vi "PECT - Scan no trigger - Autonics - each line.vi"() -> ()   [LabVIEW 2018]
uses:
  <vilib>/DAQmx/configure/timing.llb/DAQmx Timing (Sample Clock).vi
  <resource>/objmgr/daqmx.rc
  <vilib>/measure/NI_MABase.lvlib
  <vilib>/express/express analysis/Spectral/XNode/ExpressSpectralMeasurementsBlockNode.xnode
  <vilib>/express/express analysis/Spectral/Block/exnSpectralBlock spectral measurements PSD poly.vi
  <vilib>/Platform/NI_3dgraph.lvlib
  <vilib>/Instr/_visa.llb/VISA Configure Serial Port (Instr).vi
  <vilib>/Analysis/3filter.llb/Filter Passband Type.ctl
  <vilib>/Analysis/NI_AALBase.lvlib
  <vilib>/DAQmx/configure/trigger.llb/DAQmx Start Trigger (Digital Edge).vi
  <vilib>/DAQmx/read.llb/DAQmx Read (Counter U32 1Chan 1Samp).vi
  <vilib>/DAQmx/create/channels.llb/DAQmx Create Channel (CI-Count Edges).vi
  <vilib>/DAQmx/create/channels.llb/DAQmx Create Channel (AO-Voltage-Basic).vi
  <vilib>/DAQmx/create/channels.llb/DAQmx Create Channel (AI-Voltage-Basic).vi
  <vilib>/DAQmx/write.llb/DAQmx Write (Analog 1D Wfm NChan NSamp).vi
  <vilib>/DAQmx/read.llb/DAQmx Read (Analog Wfm 1Chan NSamp).vi
  <vilib>/DAQmx/read.llb/DAQmx Read (Analog 1D DBL 1Chan NSamp).vi
  <vilib>/express/express analysis/Spectral/Block/exnSpectralBlock spectral measurements PSD WFM.vi
panel:
  out "Output 2D":dbl[][](array[numeric])
  in  "Open 2":bool
  in  "Simulation":bool
  in  "Stop Scan 4":bool
  out "Record path":path=path "D:/NDTENG/Foerster/ROTOMAT/Software/Roto_1.csv" caption="selected path"
  out "Feature Extraction 2":dbl(graph)=0.021153968958947764
  in  "3D Surface":refnum<k7>(container)
  in  "Stop motor":bool
  out "Out Array":dbl[][](array[numeric])
  in  "Distance_":dbl=500.0
  in  "Right 3":bool
  in  "Left 3":bool
  out "Y line":i32 caption="Y percent"
  in  "Move X":bool
  in  "X-length":dbl=20.0
  in  "Y-length":dbl=20.0
  in  "Step Y":dbl=0.2
  in  "1 Min":dbl=0.4
  in  "2 Max":dbl=6.0
  in  "1  Max":dbl=6.0
  in  "2 Min":dbl=0.4
  in  "1 Rate":dbl=0.2
  in  "2 Rate":dbl=0.4
  in  "Travel per Pulse (mm)":dbl=0.002
  in  "Cur. Pos X":dbl=-33.28 format="%#.4f"
  in  "Cur. Pos Y":dbl=30.0 format="%#.4f"
  in  "Save Speed":bool
  in  "COM Port":refnum<visa-resource-name>="COM4"
  in  "Baud Rate":u32=9600
  in  "Data bits":u16=8 min=5 max=8 step=1
  in  "stop bits":u16(ring)=10 items=["1.0"=10, "1.5"=15, "2.0"=20]
  in  "Parity":u16(ring) items=["None", "Odd", "Even", "Mark", "Space"]
  in  "Stop Scan 2":bool
  in  "Scan 2":bool caption="Scan"
  in  "Move Distance (mm)":dbl=16.64
  in  "Counter":tag="Dev1/ctr0"
  in  "ViewMode Analysis":i32(ring) items=["cwViewXYPlane", "cwViewXZPlane", "cwViewYZPlane", "cwViewUserDefined"]
  in  "Plot style Analysis":i32(ring)=5 items=["cwLine"=1, "cwPoint"=2, "cwLinePoint"=3, "cwHiddenLine"=4, "cwSurface"=5, "cwSurfaceLine"=6, "cwSurfaceNormal"=7, "cwContourLine"=8, "cwSurfaceContour"=9]
  in  "Open":bool
  in  "Save Scan mode":bool caption="Save Process"
  in  "Tab Control 2":T1(tab)
  out "Hall sensors signal":waveform(dbl)[](graph)=[{"t0"=timestamp(3525645621.636764 s since 1904-01-01), "dt"=1.9999999999999944e-06, "Y"=array[2100 elements], "attributes"=variant("NI_ChannelName"=variant(string "Dev1/ai0"), "NI_UnitDescription"=variant(string "Volts"))}, {"t0"=timestamp(3525645621.636764 s since 1904-01-01), "dt"=1.9999999999999944e-06, "Y"=array[2100 elements], "attributes"=variant("NI_ChannelName"=variant(string "Dev1/ai0"), "NI_UnitDescription"=variant(string "Volts"))}]
  out "Feature Extraction":dbl(graph)=0.021153968958947764
  out "Waveform Graph 2":waveform(dbl)[](graph)=[{"t0"=timestamp(0 s since 1904-01-01), "dt"=1.25e-06, "Y"=array[8000 elements]}]
  out "Power spectral density":cluster{"f0":dbl, "df":dbl, "magnitude":dbl[]}[](graph)=[{"f0"=0.0, "df"=238.09523809523876, "magnitude"=[-25.4340272409559, -28.495970805276507, -69.09064054555873, -79.11355871279994, -75.69366097931027, -84.18131507822396, -80.50168881348966, -82.72314293089615, -87.19630499623688, -82.83568021481967, -89.95290866002237, -85.90392585035596, -87.41269111550386, -91.40893948681482, -86.69370819914215, -93.36336146616782, -89.019380476413, -89.73232030153878, -94.58261196624535, -89.16287927388944, -94.965890302584, -91.86846413178648, -91.95327957161693, -97.62687167891286, -91.59993648735762, -97.30685711015555, -93.8350762480425, -93.27921214218685, -99.59438563802183, -93.1824258709588, -98.3113125531512, -95.45425138584356, -94.39327135467576, -100.65352961491782, -94.55889081970952, -99.40788907105079, -97.93617495318924, -96.19517579047603, -103.97036797797732, -96.40295202889732, -99.7036956909043, -99.48760137175819, -97.46192979187015, -106.29271483151813, -97.51447379981207, -99.86179280251669, -100.43811038443037, -97.59011642740829, -105.58363666166275, -99.01126121197593, -101.01575323613292, -101.90167607549864, -98.61952569586691, -106.73670466995647, -99.29976101634999, -101.54959604687718, -105.17330050767885, -100.09392305285375, -109.78264848704497, -100.98914236173123, -101.81665207962125, -105.42358374403365, -99.82880728595141, -107.07330885402075, -101.07712607444097, -101.03780825357597, -107.32811151840846, -101.221643458408, -105.63776326231454, -101.8420593566944, -101.80081629073969, -107.47915505307212, -101.12986632760553, -106.84901404755908, -102.73715610491038, -101.51552854007832, -107.28771371003282, -101.3928633472346, -107.44515355816633, -104.89304864643535, -103.1455098860718, -110.19910428997925, -102.73063833081197, -107.57101838377707, -104.90574568581201, -103.72599931018533, -109.97178587260123, -103.24611921258705, -108.36098023558972, -106.6408311450923, -104.73569536588386, -116.21683530762306, -105.02627439976544, -107.15856030450797, -109.81191038702062, -105.53476822084077, -119.10077766590356, -105.31867536160968, -106.9718410299748, -108.34458911268797, -104.70307996109247, -114.76704583683203, -106.29948298493936, -108.55077108437321, -112.16618350190343, -105.98453547558171, -114.68576835450673, -107.50968901677987, -107.89174277914348, -111.59875709602721, -106.69368240333122, -114.93273233954758, -105.23904516482949, -106.00272331017348, -110.36103151258544, -104.93177986717492, -110.8835476773746, -106.69346348818806, -106.66103973993782, -119.11729839814336, -108.06338160849775, -114.5879267769655, -108.59816838472844, -107.53189260743514, -114.07390818184973, -106.70996756049796, -113.27381274118753, -109.50270539577696, -107.37282420343303, -113.4779718725949, -106.04267666963091, -111.30294425571472, -112.46717993668915, -109.13164915488709, -116.65287200885172, -107.03002573045511, -110.21479040603631, -112.476075561056, -106.97710947409149, -119.42145279296255, -108.3200486628316, -110.46641858585929, -117.16650627564961, -109.73297826697552, -120.31689830731365, -107.19513745371916, -110.66663569403087, -113.30365980039964, -110.01971553524372, -123.68660617105166, -110.8171755739396, -111.11382172813546, -117.76239209582961, -109.49899370205401, -115.22252846498625, -111.1932077339224, -112.38235939086871, -118.22207022901702, -110.6546796895719, -116.97450780644367, -110.82401674194465, -111.96705198878843, -118.28092956599232, -110.5621503678909, -121.25720613496851, -111.98371482341479, -113.27928013246557, -111.96833712758355, -108.56859286664552, -120.32790468431601, -110.82699792221703, -110.79062667340345, -122.65756767769517, -110.48843456045427, -116.8782055296399, -115.43719816168479, -114.47619780315773, -121.42183196132746, -111.60631415727042, -120.68077308056417, -109.35478690141552, -109.03210709352732, -120.6260555904793, -109.47936424950136, -113.33719701518146, -112.88325992990137, -110.99901978536154, -123.19636626521421, -109.09861317900774, -113.33125158106256, -115.35673297389727, -112.77249677632989, -124.61163141716472, -114.68140920359865, -121.89642913325117, -115.47413298424323, -112.82196063671608, -127.87542521315149, -111.54178118788309, -113.6448752704395, -120.76569423868874, -112.98651214877823, -123.18868565400437, -115.41399838634062, -115.46853076016815, -116.40989072804102, -110.69611347288615, -132.23164080331392, -114.76376391429793, -121.7246597336247, -117.46893009589195, -114.01899156779395, -125.22079066032327, -114.59524199183258, -114.50034890537415, -122.9532092227648, -113.72727798159212, -125.65163915514907, -113.4793801211504, -110.4090756414644, -125.63592649005872, -114.22938378193007, -116.74947251106808, -121.60535557984142, -116.79385283402802, -122.44667696630361, -113.43873413563811, -123.28159708694415, -113.92892974938164, -114.01193823589753, -121.62751955742443, -118.76839573694522, -125.52998605097204, -115.19609643487229, -117.49409595176479, -117.08423885198002, -119.48314867245172, -125.01675515413412, -117.92668164142911, -115.55962389856793, -125.63488616674975, -119.11862859365166, -114.78860770332909, -117.18339781294443, -111.18063004722558, -118.31775966044624, -111.6867367949252, -114.57226159377, -119.36541212960576, -113.90245139442648, -132.46343443313128, -120.1282759002165, -121.05279009698619, -118.9115822659523, -121.23280439248342, -116.31914159559688, -127.38829313950257, -117.34673005740623, -115.95249861902771, -114.9301657394146, -123.22361802797445, -110.83274939062106, -116.16624248562111, -116.76753364192771, -113.94454545069023, -122.95736945775944, -118.66755800656253, -129.1462641201204, -116.6351050110328, -117.22529407303742, -123.80212197360244, -115.89792176423389, -114.25823938606595, -125.60467961977515, -114.59958849364433, -121.70071005514421, -118.25968972451209, -114.69929400946009, -123.88209034116528, -115.03869272537257, -117.52034211782204, -115.27990843516797, -117.85366603932033, -125.16865559622727, -118.21960424638507, -119.69008755413566, -117.24640963460672, -114.32867295013791, -119.1576982419508, -122.85495988425586, -116.3373010103401, -114.53730203699834, -115.67017599990201, -127.144321037601, -115.73849102686786, -117.7626163106355, -119.7346592991025, -117.41317517684553, -125.0417974461613, -114.5488949833583, -116.59812516173781, -119.91064563147799, -115.27933218667663, -122.09990513751134, -120.95678574143693, -123.25641714743752, -112.5173710452192, -113.53735878806998, -129.23914933506734, -116.27157269711533, -148.4020512032711, -118.84888216023774, -123.82550527215588, -116.87770979616658, -111.32191810025745, -124.32675905891588, -114.37182733794062, -121.10713785851372, -122.59698730059695, -116.38346694563282, -121.69144349152856, -119.00883142493832, -110.81886738196273, -120.7909830607913, -115.01780448665316, -114.52055121633796, -132.6824191654361, -116.330695115645, -126.4664151018508, -118.32717907779282, -118.7288071595281, -120.42749846140066, -112.53185615773879, -124.26026008984286, -114.24089252048742, -120.00368190003405, -114.71738500842926, -112.92262025927133, -129.21127897188563, -113.5947811765517, -117.80802009651353, -117.0133790103226, -112.19210322760304, -118.17549968071762, -119.3256187825503, -118.84981507334446, -121.39118969751144, -114.64543555194373, -119.84814933224528, -114.09123407848944, -116.22899352170892, -116.41650104077173, -113.70057202673476, -124.52773908304957, -114.87372641784933, -116.11651108221098, -121.68680962246994, -115.78306007961302, -122.22621008657796, -118.81157995182392, -113.9402115821658, -132.636729517989, -114.49554876936634, -119.50980190398928, -123.27410972236837, -118.52851881066383, -122.25212982572599, -117.13947036230024, -120.85005588797962, -118.41526503460501, -117.61788553858068, -126.3872056783977, -114.98198608543298, -119.7789938911847, -120.84873579392627, -114.38831474301695, -153.35954756825245, -113.19505610638078, -114.17454820985151, -127.41069917723112, -114.92677241657191, -125.49053973810628, -113.36382196587914, -119.96785250843519, -122.47388530423243, -116.38671253508838, -120.0905790211523, -119.83326265062107, -117.88168146696918, -122.3132169880757, -115.87324909105399, -125.92003267803432, -113.96860176867415, -114.49156118371398, -127.52634390035722, -115.05967156528004, -126.82020221981517, -117.93643187259194, -116.51163213641807, -119.47551219110167, -119.55225172256931, -116.9512257852571, -122.23153124485954, -120.8368476753637, -121.48473913072222, -115.83122660909913, -135.74260014140523, -116.58358375805423, -118.15236945484727, -119.06674062398864, -115.7844834762477, -125.06111738611818, -114.7801535050972, -115.2696605691888, -123.98656374010793, -119.29025555731172, -118.29146803784099, -119.55696172158135, -118.06884171238352, -127.81587648134607, -120.41730580797976, -123.49626136731604, -112.2147141798107, -116.22555232584983, -132.79419178871254, -119.66964883124663, -117.20946469243259, -118.20939292735417, -115.6951914646649, -129.64892855822356, -114.27056999288617, -120.31005512957381, -117.41846777372632, -115.50158386260813, -124.69777160737624, -115.2892897247205, -123.61522771666871, -113.75248734362687, -113.22999749252833, -129.3490509395313, -116.88137735661701, -116.94110280242681, -119.50244079984806, -119.30521139999144, -128.17199984115797, -118.06736594940236, -116.05331575995922, -121.29670750650897, -116.1140297602044, -125.090619084802, -121.41807296062154, -120.01332757902264, -120.54914530643151, -116.49738633175463, -122.32551291835904, -118.3190808346865, -118.92638453656723, -122.48819531011718, -117.01021725424317, -120.98896352560598, -117.23831688685218, -121.27915259197124, -121.20017251921661, -117.6155648860373, -120.91300272912063, -117.94438460863424, -115.94437430101533, -123.35904829443987, -117.74011174503076, -121.54935745388448, -120.82564553545025, -121.98951430455743, -120.24858103448778, -116.44403527138395, -112.79571494351876, -112.42801913096545, -110.1697573019791, -115.34500457736401, -119.81921052956707, -129.82600951154313, -115.5862301263047, -112.59292882433087, -120.79009137478283, -131.32849293387295, -113.61194478398238, -123.48568856527031, -119.17507777781304, -123.09261867490484, -116.97755217417308, -123.94453461434183, -116.58080525616379, -119.64289646280756, -122.90202645580743, -126.66219093058154, -121.95048829056148, -115.72578023509817, -116.70117814464484, -121.91050280869723, -118.25299095698178, -116.45905559047064, -132.57794493731578, -121.65327820443292, -120.9816664775787, -117.17270262269045, -120.27433984830965, -125.89418976028173, -119.09563505847817, -126.9693215534833, -113.17465524665704, -118.98702092883116, -119.83822568580342, -120.45832738089722, -120.67735960513633, -127.38676010839353, -127.65777338183055, -118.37446329057411, -115.61355494839711, -119.94568688114103, -116.06619937633681, -126.348857777089, -118.92850079147068, -119.5416617639739, -132.47075644221843, -118.08809356028496, -123.16186463092723, -121.51579486791232, -122.88983670053283, -129.5195538417256, -120.4730389608841, -132.16486858341602, -122.34690358436781, -120.71922104337597, -114.29260860841114, -117.67902631803368, -124.7040155514909, -123.51274592117205, -120.02297921674332, -136.54655493811157, -120.45629227407751, -119.06410204276258, -127.91681714792554, -122.82090055753153, -125.16838176650813, -121.79565386970478, -119.79607311590995, -126.54861375039647, -121.59135878113302, -132.8348640697562, -118.1305434733294, -120.46070148841905, -122.69571910896963, -117.6534954653865, -124.15742546824006, -120.73646926947502, -124.82696993800742, -124.513836786494, -123.15395713389651, -124.62395468806395, -117.21365768658171, -119.32635871968456, -121.48532284413152, -119.38242892643675, -126.25575652510352, -123.27133124029851, -117.58533922728374, -118.17710108929799, -114.99496360200965, -117.77133194647278, -111.34898201101595, -111.50817058307922, -119.0703124690998, -127.70676079885351, -121.8704969141074, -125.93154214283446, -118.65628450081473, -122.47918878348962, -117.9651589546518, -126.13560583004508, -122.42294805637847, -133.924453763793, -117.2082573038767, -117.6525335446734, -122.92077297426977, -122.04624645756786, -116.43289028226238, -117.93180959338378, -129.02356734231915, -117.95493621286326, -120.7555929766252, -120.76782849311112, -123.06287498470708, -117.83798593857965, -123.43423215434719, -120.15190119516652, -120.48240443128407, -143.29738987393452, -123.46572247444769, -120.89055325172792, -125.66715973809033, -118.26887578998644, -117.01836200028421, -121.33021830755509, -119.68846363313813, -122.60689066103069, -116.26858138914181, -119.59360791972998, -122.94866175463353, -114.174409515556, -118.00516930888391, -121.56978543579633, -135.87799017759036, -117.50816594504829, -122.82539428457626, -123.82103443155845, -124.77975840345442, -121.13340798086698, -120.93607435603558, -133.15787160745222, -120.70545628137863, -125.02155972441679, -122.04666465472178, -118.01234649746348, -127.88767491042842, -119.02096620167217, -120.16031065152875, -122.25406107859625, -121.72733059051095, -120.61357375519918, -118.63962847172827, -134.3857741605498, -116.3600853185034, -117.26695700691671, -119.9176982185873, -113.45576465218444, -126.69779573632724, -114.39554522802246, -116.8457146515868, -116.34219889483086, -119.30011291548334, -120.01163291843496, -114.29497178248809, -127.65687642749229, -119.58556923753022, -129.8593054181261, -122.2353645100479, -120.79536520223796, -119.83284028355028, -117.7991246185715, -128.390292904734, -119.78079925213122, -125.478913448993, -113.89747777944768, -112.66620124153357, -124.3475049842711, -120.85847303094337, -132.91807981902295, -119.523494985723, -116.65149909866443, -119.73287290436721, -127.63237851524192, -127.23413304048789, -120.87585453904362, -121.08540368080186, -134.91071939669257, -117.75375801669338, -117.2683014590723, -120.9739099492833, -118.23809733632451, -120.94065804928206, -123.88077510875804, -118.13812819300607, -122.60294123365466, -126.97075898006995, -120.18754789731035, -124.71238663441227, -120.55456557278582, -130.94599087480253, -111.18288669417035, -112.27708791831247, -126.0512034600378, -117.41881712783596, -128.20553880273903, -117.29482600885808, -118.2045526390752, -127.81966672699878, -117.03716165902529, -115.46711739757512, -117.15363929234843, -121.87599671671335, -121.19736800869221, -126.5301786755875, -131.20754947382918, -124.40138004810741, -129.0562496906515, -121.06816554587536, -121.01023627802867, -138.6137911215848, -120.12495002524031, -121.38510517514229, -122.79804220535513, -116.97501378195477, -118.82011581137473, -114.0229185604644, -119.54287501990726, -114.64474566771625, -117.76935669872461, -123.81082574158907, -118.51678358865587, -128.9664755188374, -123.45357998434133, -122.74888841574231, -120.74640581234044, -126.956344345126, -119.95682140104577, -118.8873101779055, -124.41062359284174, -128.97304498664363, -123.86287113204068, -127.30257087528216, -120.61364220528216, -114.45119129304715, -119.68384044686806, -131.29639185291157, -122.31250766293485, -119.57420865241102, -124.74014026002448, -124.87593035709094, -118.4566565612952, -123.76236085976001, -120.84780538841838, -117.68987599773281, -135.06195695255914, -122.56143585795171, -129.04610316842883, -118.32313199570537, -117.77093802786419, -124.46572845786741, -129.1123298336903, -120.88470269965448, -116.69988985752187, -116.84054667499878, -133.76883696987278, -122.32434984927302, -124.98940594457933, -122.56515592789917, -118.31562562243366, -133.97049179545627, -122.33220627999802, -131.16753675316977, -124.69828063969263, -116.37621154460467, -126.1833423168025, -129.62937634161355, -118.46241371150788, -117.52851478852457, -125.32425037236442, -119.0327364293772, -124.2861355894013, -123.24573502278234, -125.52155812053758, -113.75743410709823, -114.79513162658353, -128.58142362588052, -122.48277095196701, -118.94747544412269, -123.86988127835491, -124.78140456983323, -121.53998481875398, -116.01432822539552, -119.20174681160661, -122.75167725800814, -120.58657749420254, -118.51141061842183, -119.24457006171983, -131.43641234223372, -116.00759139055087, -121.24442216102587, -123.29371279953725, -117.608355420454, -116.33684374617326, -118.06291688281922, -121.88761866022774, -121.54820313120047, -119.5051369873635, -126.56611158390913, -118.84012713615805, -121.09285296522563, -124.67955377692547, -147.31451139022337, -116.80660421066897, -114.8367853755961, -120.41026468628925, -123.65666101895222, -119.64837119787269, -116.77480172559095, -116.54263359173909, -124.75286620868079, -117.33721912698883, -116.51795620907136, -118.50086748176733, -128.10381328920522, -122.78098994574157, -120.24716756092855, -119.52743204722819, -115.00407387659232, -108.2853711552629, -108.61086943894702, -119.6228894146785, -124.11132022420912, -125.6202218409766, -123.1749360787656, -118.1971196161698, -123.95075368058998, -121.72140109898365, -123.27106899042522, -123.73035629887062, -121.24369679109273, -121.07381526465288, -113.13965659723667, -118.330755475899, -118.40249076804484, -111.59630598649044, -116.1569506845575, -125.67326089915758, -125.85723567111906, -119.24293277595024, -117.87067617433537, -120.70936924059559, -131.8090588468898, -132.98711569625004, -123.63274249467587, -122.75476917502559, -126.12873814250243, -120.53144270605179, -129.07030822919336, -122.7889410422919, -124.35405971166259, -119.63968579420454, -139.0154441054289, -129.47962001806934, -121.86548015410847, -128.6818469257012, -121.40195873232601, -138.64231053781285, -124.22025721762265, -124.06073958736941, -126.71929802352521, -131.7498459276443, -120.68144109742178, -122.6325588818875, -126.80796617875095, -124.92487955227033, -136.94498040498806, -124.26704334219014, -123.21376211221711, -140.25352033075964, -129.53222319772195, -122.58541579060463, -122.1996729592375, -125.66642108013673, -125.66310429236694, -120.09682773706965, -125.27326633941439, -121.55721878725502, -121.22507119941083, -121.53716878624485, -136.20685498111987, -128.15260146013156, -120.03473972471616, -124.60755958763912, -124.73082500077143, -123.93425949983688, -131.04483249265184, -121.7957035014449, -127.09321441816094, -133.6144579272493, -124.69014595896968, -130.4902091211609, -121.18031440773905, -128.00033943961677, -125.88991118115149, -118.865310745079, -123.69668867733147, -117.98756965862728, -114.40013091842827, -118.28685032521078, -122.23464196869948, -124.8440422629961, -129.66281606870848, -119.440534215621, -124.54391783563877, -124.93447967158188, -121.7258558761523, -122.28817885403082, -127.06889620458577, -128.92172974939206, -120.62932166634072, -126.06847321900452, -123.31471168429935, -121.80350826545656, -129.2574604322076, -125.67225933193998, -125.7801671825605, -129.53804733161627, -119.56756644124712, -128.82490314699373, -124.7689736295626, -120.50019729114693, -124.50603158563972, -122.8120627011088, -125.60528875555717, -123.8817354922713, -124.05570537836674, -120.94568834491936, -118.06056028605255, -124.24390361274648, -125.5716703018188, -127.71949519914061, -130.7001652968252, -126.27701412017494, -133.76810134709916, -128.4738939614179, -120.302550881701, -118.91298143662928, -124.9077318110765, -127.16253699189492, -118.11405934812818, -117.52028071290711, -140.95620572748925, -123.61977932545628, -131.0334379970501, -125.88948384968432, -127.81552331993379, -121.92316280719056, -119.05911238768732, -126.83773251459189, -123.52627415002164, -120.8779561023192, -123.66683567603742, -131.64300993967345, -123.62895847772963, -116.89792951363142, -120.1068259250195, -117.92484706459337, -115.58208487778379, -120.76803581628594, -123.95408562090736, -122.79456549632754, -134.5305398779298, -123.57040300991032, -128.40634159414552, -123.70102187824159, -118.24970739397313, -119.66483900349026, -127.78024313111393, -120.3547204111785, -125.49305364308705, -119.49505591004302, -120.50920386196539, -119.03509516851003, -114.24667300009652, -121.60538636584391, -119.95304417598024, -122.24585853682832, -128.63653016912684, -116.04810628805795, -121.94159862131235, -122.59928204398939, -121.4532410501923, -128.6511474663462, -130.83715595958148, -121.71998300574741, -116.91426629511156, -113.587592058512, -115.59736707638731, -124.65300822631244, -133.32538684258748, -124.02289142873636, -121.54278890993639, -119.02596809402394, -108.90572887117857, -112.14974069608851, -129.21149299565423, -118.82148342951197, -116.65510894288538, -118.39609618084175, -116.53502642884725, -122.47549439965209, -122.23125657046063, -123.68081343116663, -120.67915071600007, -123.6899360128769, -118.56721985209728, -118.36641581191942, -126.96724630704657, -119.36877661672403, -123.07698921198843, -117.80772421906035, -122.82545076270567, -118.82755071380888, -117.21030132539394, -129.760567864525, -118.0816708063509, -125.80573274113647, -121.18434666182338, -121.80987210832065, -130.99259828357094, -125.47223579895922, -123.86818606677002, -118.7118158196511, -119.27778317338742, -127.27333258839096, -119.90672352079164, -140.78772370844268, -118.08251080057329, -119.86636232122572, -118.69482489738232, -119.19106512767372, -123.70988914879189, -121.92566832147995, -123.41378261726373, -120.1715186070818, -117.9079629421116, -117.41960207545632, -123.72833996166874, -127.24377206607298, -124.99098647980887, -129.48803701799955, -129.92351350561592, -120.79284154834647, -119.29601975194524, -136.17244775530037, -126.73975437546255, -128.84068276143336, -125.66374985701982, -136.69026010435715, -125.44409235146617, -119.28138070315057, -118.65017329869724, -118.02521532826772, -122.23736063759657, -121.27846943548622, -116.69850478126861, -119.7711336696722, -123.70776561180185, -118.43344549561263, -123.92390877157247, -117.19637143066551, -117.64112988205311, -127.78399195238529]}, ...(2 in all)]
  out "Differential data":dbl[][](graph)
  out "Normal data":dbl[][](graph)
  in  "Emergency Stop":bool
  in  "Stop 3":bool
  in  "Home Y":bool
  in  "Home X":bool
  in  "Back":bool
  in  "Front":bool
  in  "Left":bool
  in  "Right":bool
  in  "Stop Scan":bool
  in  "Scan":bool
  in  "Tab Control":enum32{"     Motor    ", "         DAQ        "}(tab)
  in  "Left_":bool
  in  "Right_":bool
  in  "Home":bool
  in  "Move Distance (mm) 2":dbl=20.0
  in  "Speed":dbl=10.0
  out "Current  Position (mm)":dbl format="%#_4g"
  in  "COM Port 2":refnum<visa-resource-name>="COM3"
  in  "Baud Rate 2":u32=57600
  in  "Stop Scan 3":bool
  in  "Multiplier":dbl=10.0
  in  "Travel per  Pulse":dbl=0.0025
  in  "Low Cutoff Freq":dbl=50.0
  out "Actual Sample Rate":dbl=500000.0 format="%0.2f"
  in  "Physical Channel":tag="Dev5/ai0"
  in  "Min Voltage":dbl=-10.0
  in  "Max Voltage":dbl=10.0
  in  "Terminal Configuration":i32(ring)=10083 items=["default"=-1, "RSE"=10083, "NRSE"=10078, "Differential"=10106, "Pseudodifferential"=12529]
  in  "Sample Clock Source 2":tag="OnboardClock"
  in  "Sample Rate":dbl=500000.0
  out "Number of Samples 2":i32=1000
  out "Actual Sample Rate 2":dbl=800000.0 format="%0.2f"
  in  "Physical Channel(s)":tag="Dev5/ao1"
  in  "Min Voltage 2":dbl=-10.0
  in  "Max Voltage 2":dbl=10.0
  in  "Sample Clock Source":tag="OnboardClock"
  in  "Sample Rate 2":dbl=800000.0
  in  "Number of Samples":i32=8000
  in  "Offset":bool
  in  "2 Plots":bool
  in  "Edge":i32(ring)=10280 items=["Rising"=10280, "Falling"=10171]
  in  "Digital Trigger Source":tag="/Dev5/PFI0"
  in  "Average":i32=10
  in  "Duty cycle %":dbl=50.0 format="%#.2f"
  in  "Stop":bool
  in  "Output Array":T2(array[cluster])=[{"Waveform Type"=2, "Amplitude"=10.0, "Frequency"=1000.0}] {"Frequency" format="%0.2p"; "Amplitude" format="%0.2p"; "Waveform Type" items=["Sine Wave", "Triangle Wave", "Square Wave", "Sawtooth Wave"]}
  # "Pulse Shape"
  # "COM  Setting"
  # "Trigger Settings"
  # "Data Processing"
  # "Speed  Setting"
  # "Scan  Setting"
  # "Pulse"
  # "Hall Sensors Signal"
  # "Feature Extraction"
  # "Power Spectal Density"
  # "COM  Setting"
  # "Scan  Setting"
  # "Pulse  Channel"
  # "Pulse  Timming"
  # "Sensor  Channel"
  # "DAQ Timming"
  # "Logging Settings"
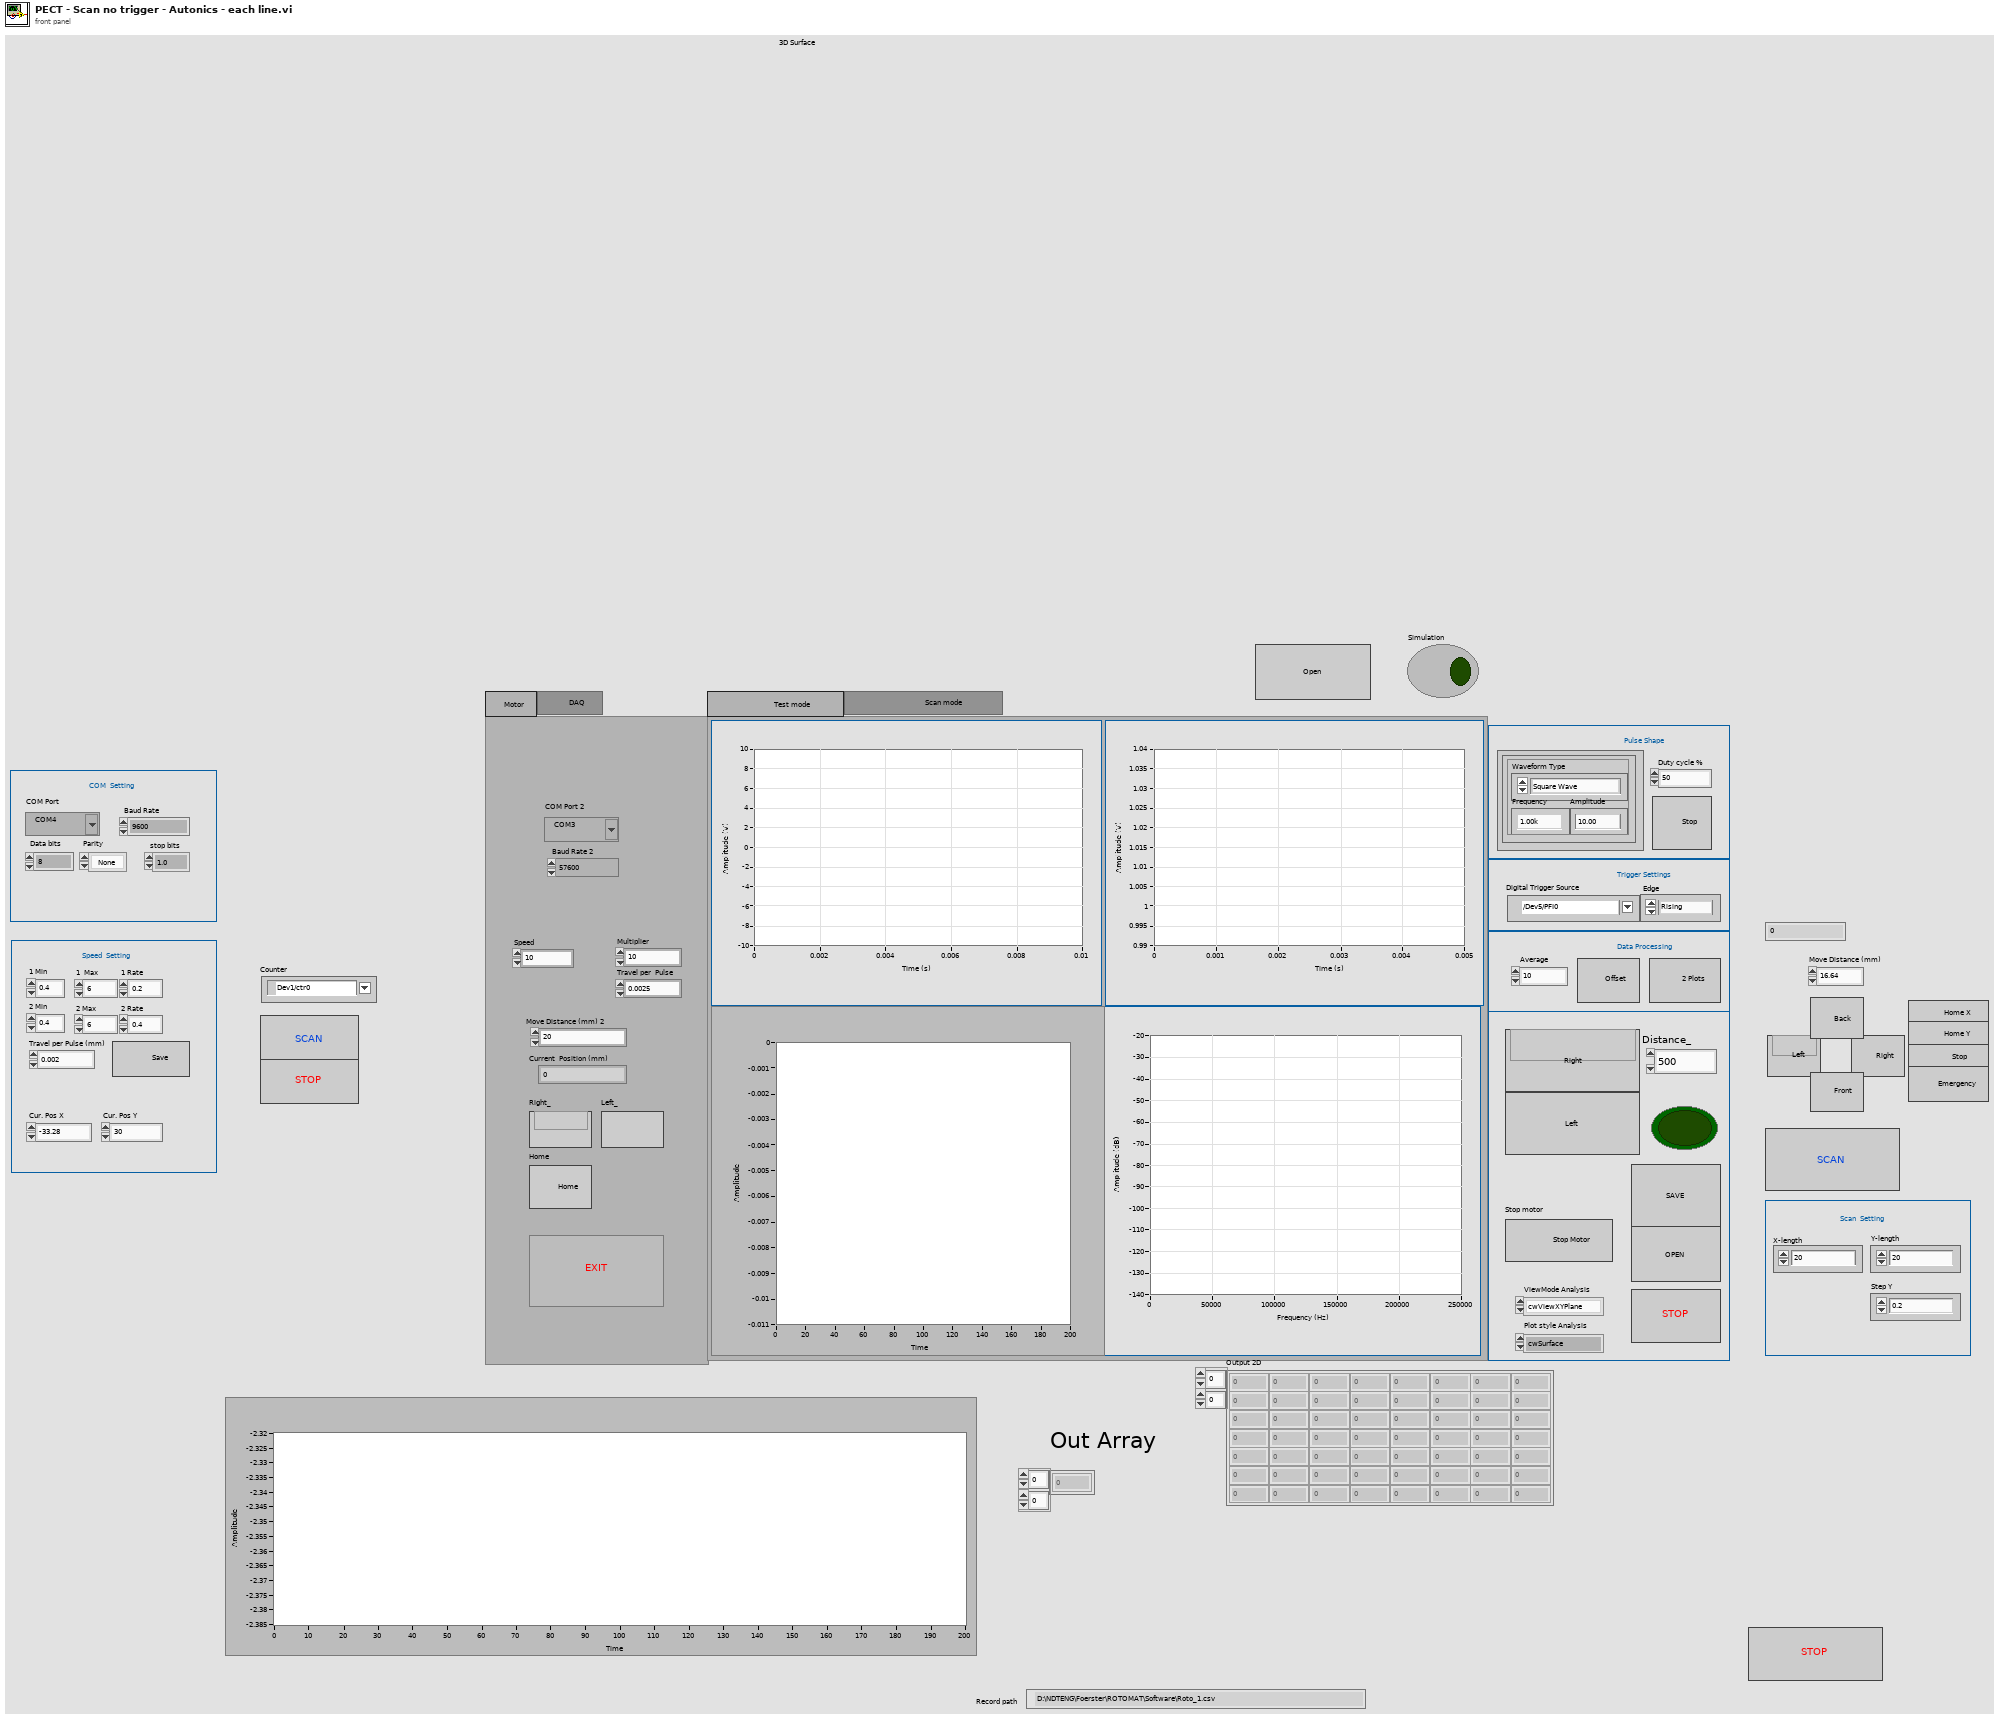
[diagram p1: front panel]
types:
  T1 = enum32{"                    Test mode                   ", "                          Scan mode                      "}
  T2 = cluster{"Waveform Type":u16, "Amplitude":dbl, "Frequency":dbl}[]
  T3 = enum16{"No Scan", "Scan X", "Wait to destination X"}
  T4 = cluster{"Waveform Type":u16, "Amplitude":dbl, "Frequency":dbl}
  T5 = enum16{"open", "open or create", "create or replace", "create", "open (read-only)"}
  T6 = typedef "NI_AALBase.lvlib/Filter Passband Type.ctl" = enum32{"Lowpass", "Highpass", "Bandpass", "Bandstop"}
  T7 = cluster{"averaging mode":u16, "weighting mode":u16, "number of averages":u32}
  T8 = cluster{"dB On (F)":bool, "unwrap phase (F)":bool, "convert to degree (F)":bool}
  T9 = typedef "NI_Matrix.lvlib/RealMatrix.ctl" = dbl[][]
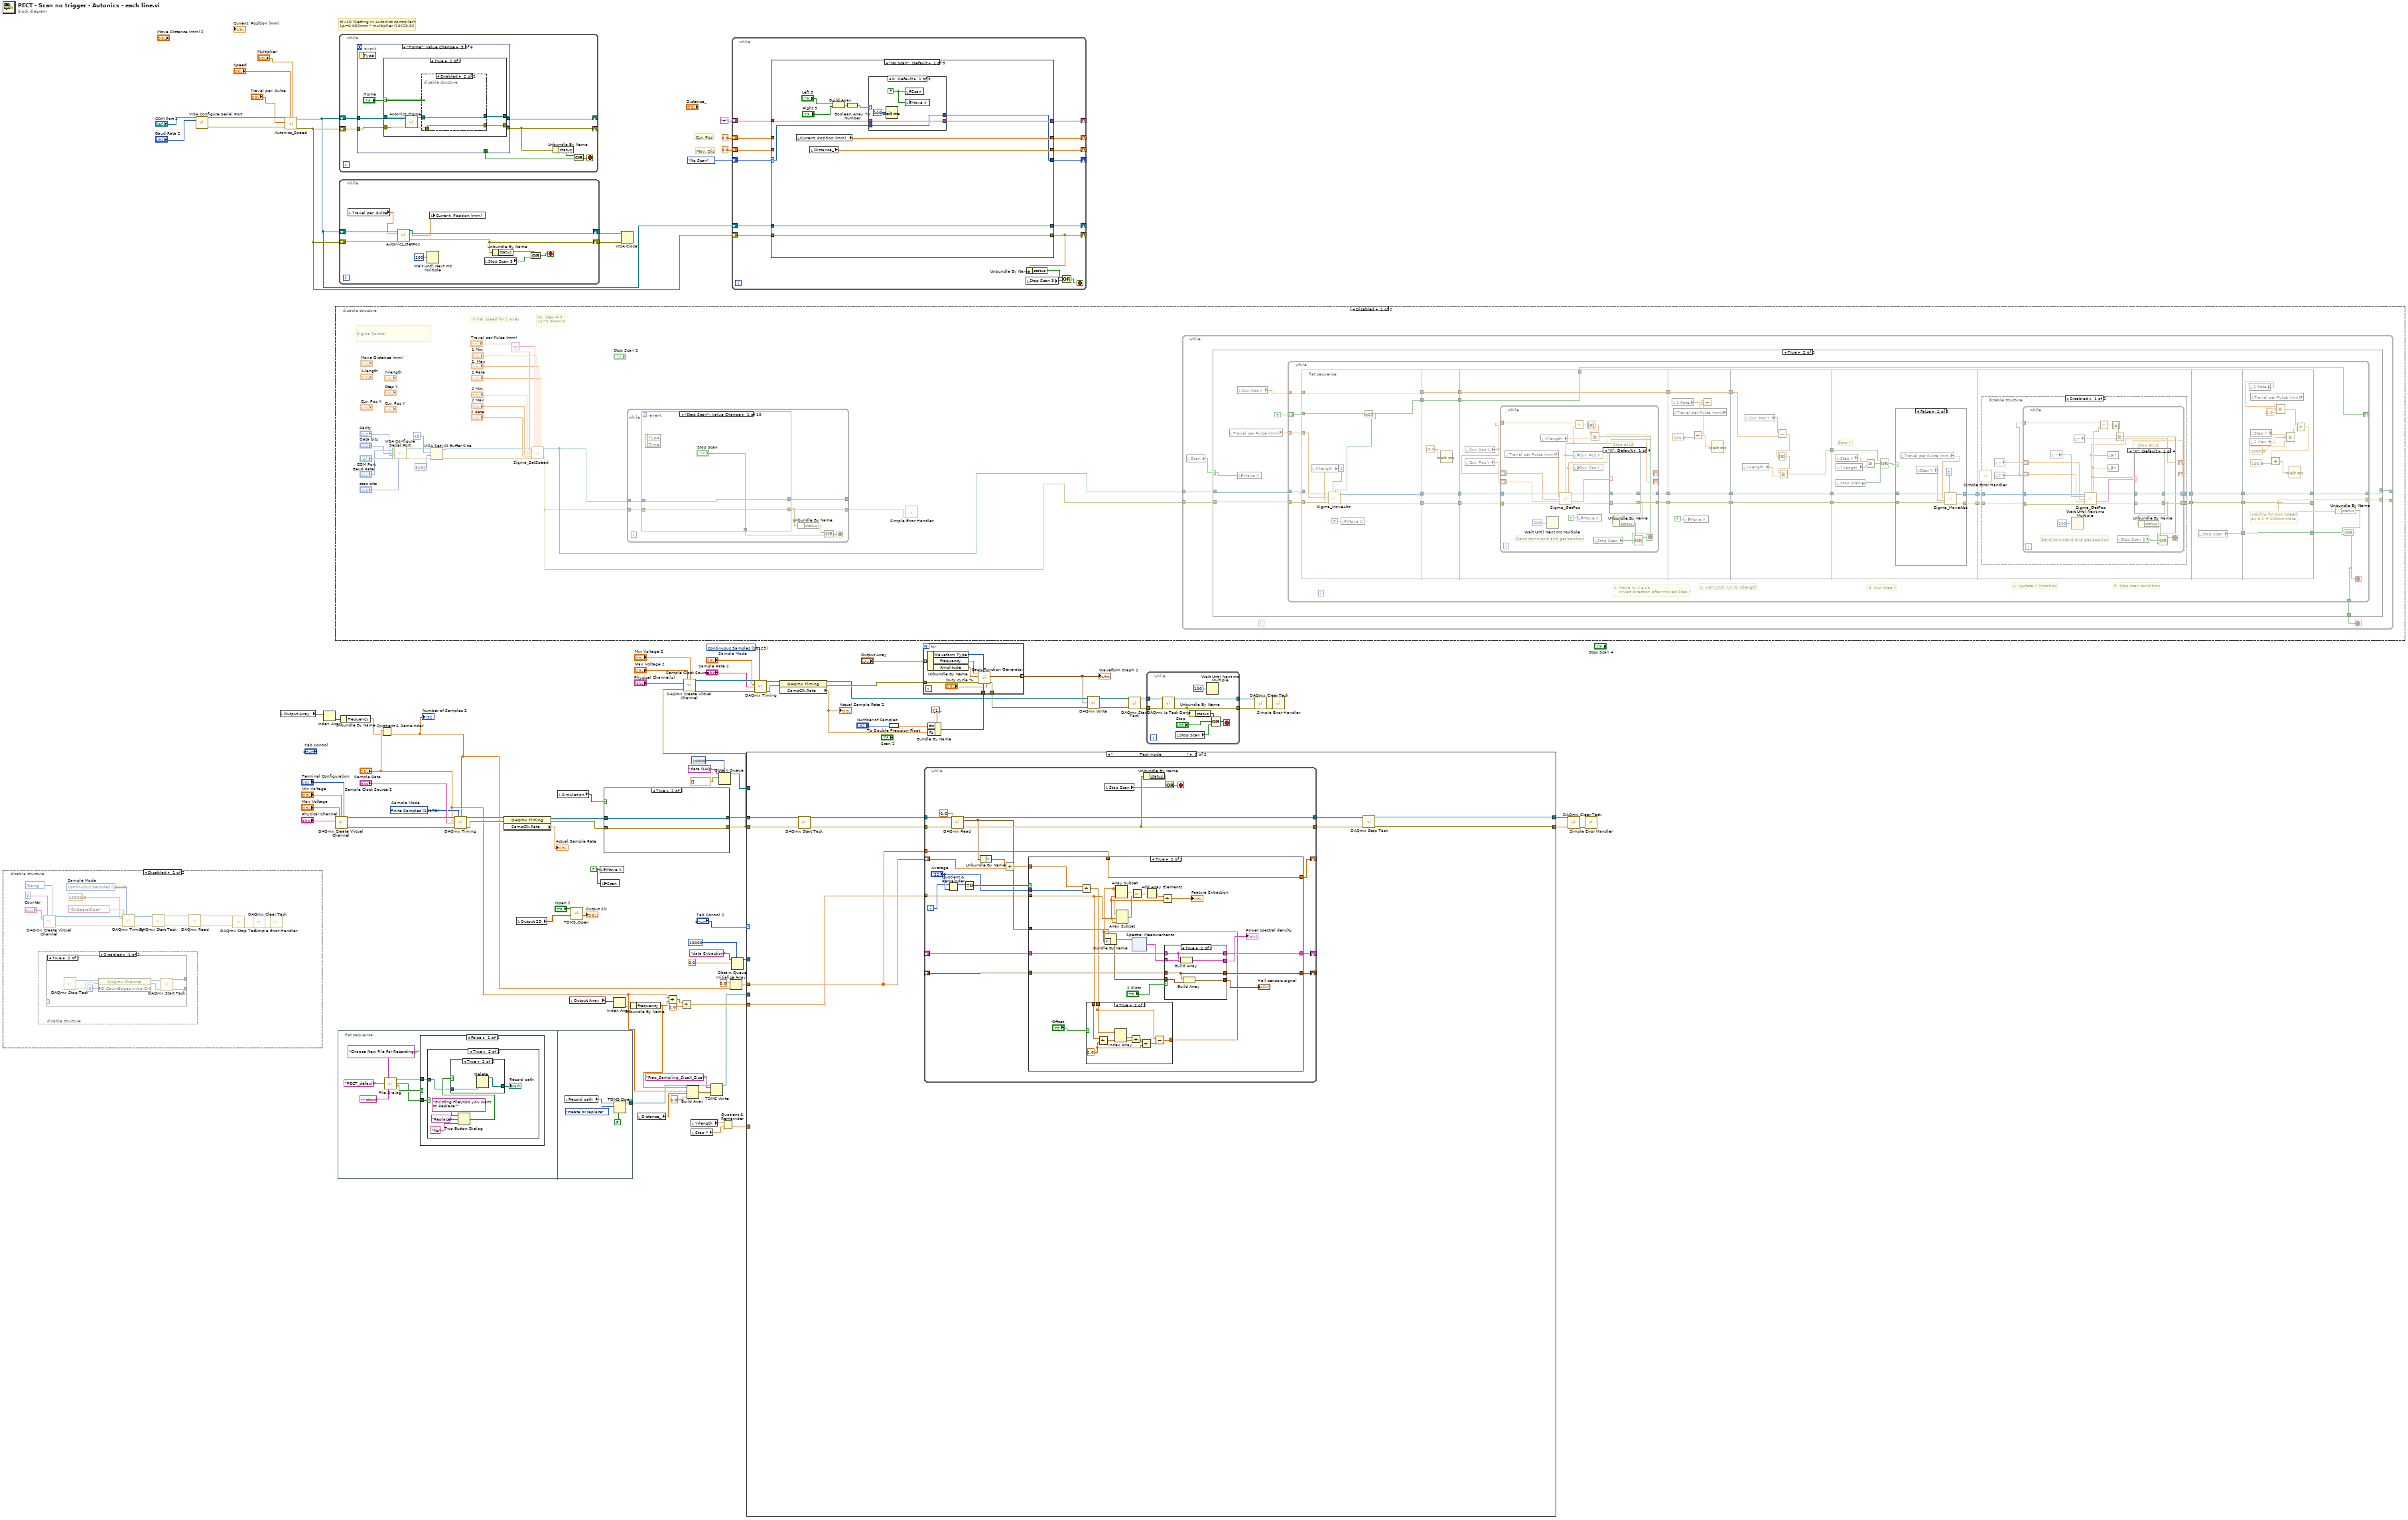
[diagram p0: block diagram]
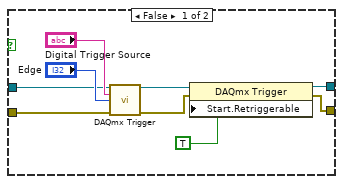
[diagram p2: hidden frame]
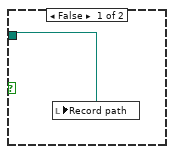
[diagram p3: hidden frame]
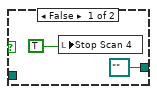
[diagram p4: hidden frame]
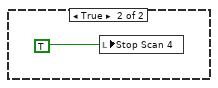
[diagram p5: hidden frame]
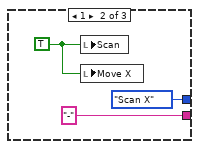
[diagram p6: hidden frame]
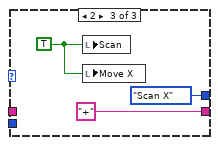
[diagram p7: hidden frame]
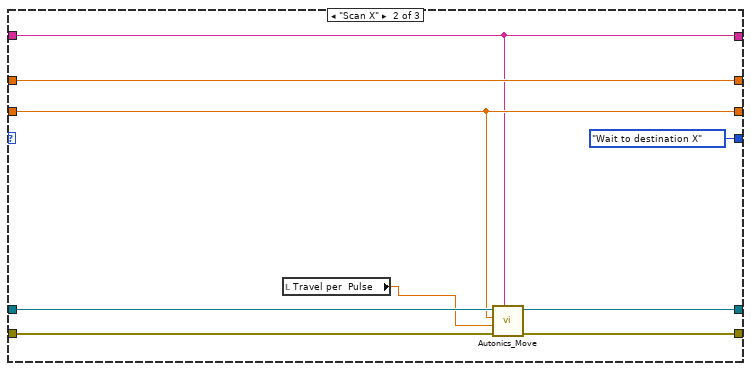
[diagram p8: hidden frame]
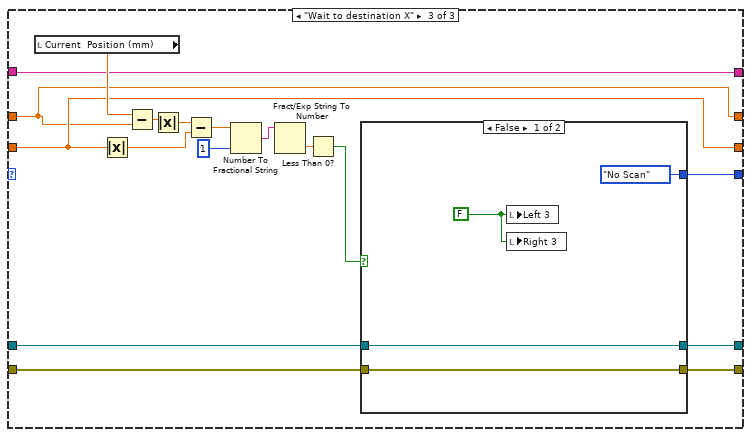
[diagram p9: hidden frame]
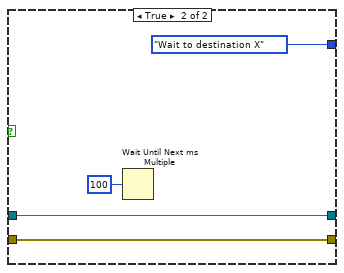
[diagram p10: hidden frame]
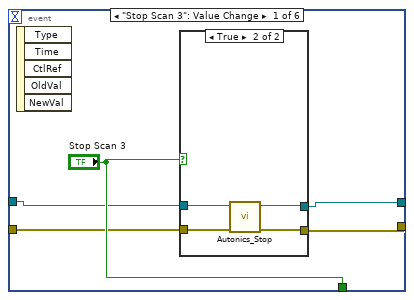
[diagram p11: hidden frame]
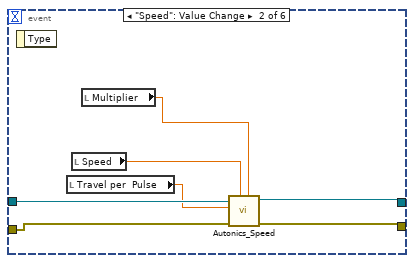
[diagram p13: hidden frame]
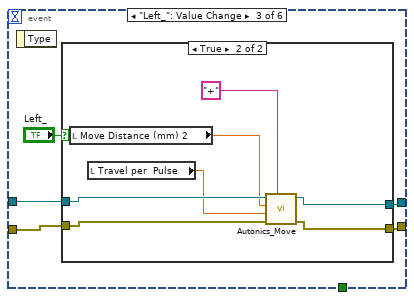
[diagram p14: hidden frame]
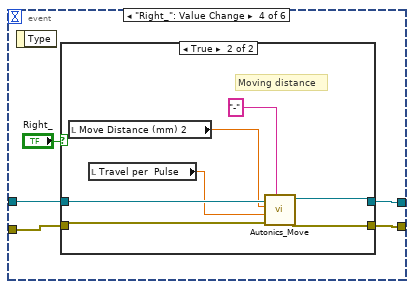
[diagram p16: hidden frame]
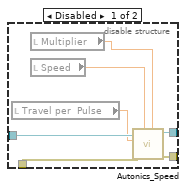
[diagram p19: hidden frame]
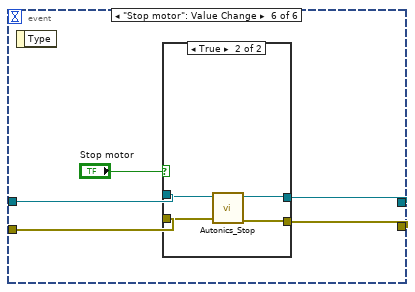
[diagram p20: hidden frame]
diagram:
  w34 = FALSE ("Move X")
  w58 = 10178 items=["Finite Samples"=10178, "Continuous Samples"=10123, "Hardware Timed Single Point"=12522]  # Sample Mode
  w81 = 10123 items=["Finite Samples"=10178, "Continuous Samples"=10123, "Hardware Timed Single Point"=12522]  # Sample Mode
  # "Mov. Dis"
  # "Cur. Pos"
  # "div10 (Setting in Autonics controller):\n1p~0.002mm * multiplier (10)=0.02"
  n1 = disable-structure shown="Disabled" {
    frame Disabled {
      w111 = 10280 items=["Rising"=10280, "Falling"=10171] ("edge")
      w110 = 10123 items=["Finite Samples"=10178, "Continuous Samples"=10123, "Hardware Timed Single Point"=12522]  # Sample Mode
      n2 = disable-structure shown="Disabled" {
        frame Disabled {
          n3 = case shown="True" {
            selector: _ -> [_ _]
            tunnel: [_ w116] -> _
            tunnel: [_ w113] -> _
            frame False {
            }
            frame True {
              n4 = call <vilib>:"DAQmx Stop Task.vi"() -> ("task out"=w118:refnum<k21>, "error out"=w115:errorcluster)  [unwired: 14 in]
              n5 = property class="DAQmx Channel"(reference=w118, error in=w115, "CI.CountEdges.InitialCnt"=u32 0) -> (reference out=w117:refnum<k21>, error out=w114:errorcluster)
              n6 = call <vilib>:"DAQmx Start Task.vi"("task/channels in"=w117, "error in"=w114) -> ("task out"=w116:refnum<k21>, "error out"=w113:errorcluster)  [unwired: 12 in]
            }
          }
        }
        frame Enabled {
        }
      }
      n7 = call-poly <vilib>:"DAQmx Create Virtual Channel.vi"("initial count"=u32 0, "edge"=w111, "counter"="Counter") -> ("task out"=w106:refnum<k21>, "error out"=w105:errorcluster)  [unwired: 11 in]
      n8 = call-poly <vilib>:"DAQmx Timing.vi"("task/channels in"=w106, "sample mode"=w110, "rate"=10000.0, "source"=tag "OnboardClock", "error in"=w105) -> ("task out"=w108:refnum<k21>, "error out"=w107:errorcluster)  [unwired: 9 in]
      n9 = call <vilib>:"DAQmx Start Task.vi"("task/channels in"=w108, "error in"=w107) -> ("task out"=w100:refnum<k21>, "error out"=w98:errorcluster)  [unwired: 12 in]
      n10 = call-poly <vilib>:"DAQmx Read.vi"("task/channels in"=w100, "error in"=w98) -> ("task out"=w99:refnum<k21>, "error out"=w97:errorcluster)  [unwired: 11 in, 1 out]
      n11 = call <vilib>:"DAQmx Stop Task.vi"("task/channels in"=w99, "error in"=w97) -> ("error out"=w102:errorcluster)  [unwired: 12 in, 1 out]
      n12 = call <vilib>:"DAQmx Clear Task.vi"("error in"=w102) -> ("error out"=w101:errorcluster)  [unwired: 14 in]
      n13 = call <vilib>:"Simple Error Handler.vi"("error in (no error)"=w101) -> ()  [unwired: 4 in, 5 out]
    }
    frame Enabled {
    }
  }
  n14 = call-poly "VISA Configure Serial Port"("VISA resource name"="COM Port 2", "baud rate (9600)"="Baud Rate 2") -> ("VISA resource name out"=w28:refnum<visa-resource-name>, "error out"=w27:errorcluster)  [unwired: 12 in]
  n15 = local read "Output Array"() -> (w4:T2)
  n16 = call "Autonics_Speed.vi"("Multiplier"="Multiplier", "Speed (mm/s)"="Speed", "error in (no error)"=w27, "Travel per  Pulse"="Travel per  Pulse", "VISA resource name"=w28) -> ("error out"=w24:errorcluster, "VISA resource name out"=w25:refnum<visa-resource-name>)  [unwired: 5 in]
  n17 = Index Array(array=w4) -> (element=w5:T4)  [unwired: 1 in]
  n18 = call-poly <vilib>:"DAQmx Create Virtual Channel.vi"("maximum value"="Max Voltage", "minimum value"="Min Voltage", "input terminal configuration"="Terminal Configuration", "physical channels"="Physical Channel") -> ("task out"=w93:refnum<k21>, "error out"=w94:errorcluster)  [unwired: 10 in]
  n19 = disable-structure shown="Disabled" {
    frame Disabled {
      # "No. step = 5\n1p~0.004mm"
      # "Initial speed for 2 axes"
      # "Sigma Control"
      n20 = call-poly "VISA Configure Serial Port"("VISA resource name"="COM Port", "baud rate (9600)"="Baud Rate", "data bits (8)"="Data bits", "parity (0:none)"="Parity", "stop bits (10: 1 bit)"="stop bits") -> ("VISA resource name out"=w128:refnum<visa-resource-name>, "error out"=w122:errorcluster)  [unwired: 9 in]
      n21 = VISA Set I/O Buffer Size(VISA resource name=w128, mask (16)=48, size (4096)=u32 8192, error in (no error)=w122) -> (VISA resource name out=w132:refnum<visa-resource-name>, error out=w131:errorcluster)
      n22 = call "Sigma_SetSpeed.vi"("VISA resource name"=w132, "Travel per Pulse (0.004mm)"="Travel per Pulse (mm)", "Min (1mm) 2"="2 Min", "Max (2mm) 2"="2 Max", "Rate (1mm) 2"="2 Rate", "error in (no error)"=w131, "Axis (1)"="W", "Min (1mm)"="1 Min", "Max (2mm)"="1  Max", "Rate (1mm)"="1 Rate") -> ("VISA resource name out"=w121:refnum<visa-resource-name>, "error out"=w120:errorcluster)  [unwired: 8 in]
      n23 = while {
        tunnel: w121 -> [w403]
        tunnel: [w398] -> _
        tunnel: w120 -> [w402]
        tunnel: [w400] -> w141
        stop <- w399 stop-if-true
        n24 = event shown="[0] \"Stop Scan\": Value Change" {
          selector: _ -> [_ _ _ _ _ _ _ _ _ _]
          dyn-events: _ -> [_ _ _ _ _ _ _ _ _ _]
          timeout: _ -> [_ _ _ _ _ _ _ _ _ _]
          tunnel: w403 -> [w405 w418 w421 w436 w451 w466 w483 w495 w505 w517]
          tunnel: w402 -> [w404 w415 w420 w435 w450 w465 w482 w494 w504 w516]
          tunnel: [w405 w417 w423 w438 w453 w468 w480 w493 w507 w519] -> w398
          tunnel: [w404 w416 w422 w437 w452 w467 w479 w492 w506 w518] -> w400
          tunnel: ["Stop Scan" _ _ _ _ _ _ _ _ _] -> w397
          event "Stop Scan": Value Change {
            n25 = event-data() -> ()  [unwired: 1 in, 2 out]
          }
          event "Save Speed": Value Change {
            n26 = event-data() -> ()  [unwired: 1 in, 5 out]
            n27 = local read "Travel per Pulse (mm)"() -> (w407:dbl)
            n28 = local read "1  Max"() -> (w412:dbl)
            n29 = local read "1 Rate"() -> (w411:dbl)
            n30 = local read "2 Rate"() -> (w408:dbl)
            n31 = local read "2 Max"() -> (w409:dbl)
            n32 = local read "1 Min"() -> (w413:dbl)
            n33 = local read "2 Min"() -> (w410:dbl)
            n34 = call "Sigma_SetSpeed.vi"("VISA resource name"=w418, "Travel per Pulse (0.004mm)"=w407, "Min (1mm) 2"=w410, "Max (2mm) 2"=w409, "Rate (1mm) 2"=w408, "error in (no error)"=w415, "Axis (1)"="W", "Min (1mm)"=w413, "Max (2mm)"=w412, "Rate (1mm)"=w411) -> ("VISA resource name out"=w417:refnum<visa-resource-name>, "error out"=w416:errorcluster)  [unwired: 8 in]
          }
          event "Right": Value Change {
            n35 = event-data() -> ()  [unwired: 1 in, 1 out]
            n36 = case shown="True" "Right" {
              tunnel: [w425 w431] -> w423
              tunnel: [w424 w430] -> w422
              tunnel: w421 -> [w425 w433]
              tunnel: w420 -> [w424 w432]
              frame False {
              }
              frame True {
                n37 = local read "Travel per Pulse (mm)"() -> (w427:dbl)
                n38 = local read "Move Distance (mm)"() -> (w426:dbl)
                n39 = call "Sigma_MoveAbs.vi"("Direction (+)"=FALSE, "Axis (1)"=1, "error in (no error)"=w432, "Travel (1mm)"=w426, "Travel per Pulse (0.004mm)"=w427, "VISA resource name"=w433) -> ("error out"=w430:errorcluster, "VISA resource name out"=w431:refnum<visa-resource-name>)  [unwired: 4 in]
              }
            }
          }
          event "Left": Value Change {
            n40 = event-data() -> ()  [unwired: 1 in, 1 out]
            n41 = case shown="True" "Left" {
              tunnel: [w440 w447] -> w438
              tunnel: [w439 w446] -> w437
              tunnel: w436 -> [w440 w448]
              tunnel: w435 -> [w439 w445]
              frame False {
              }
              frame True {
                n42 = local read "Travel per Pulse (mm)"() -> (w442:dbl)
                n43 = local read "Move Distance (mm)"() -> (w441:dbl)
                n44 = call "Sigma_MoveAbs.vi"("Direction (+)"=TRUE, "Axis (1)"=1, "error in (no error)"=w445, "Travel (1mm)"=w441, "Travel per Pulse (0.004mm)"=w442, "VISA resource name"=w448) -> ("error out"=w446:errorcluster, "VISA resource name out"=w447:refnum<visa-resource-name>)  [unwired: 4 in]
              }
            }
          }
          event "Front": Value Change {
            n45 = event-data() -> ()  [unwired: 1 in, 1 out]
            n46 = case shown="True" "Front" {
              tunnel: [w455 w461] -> w453
              tunnel: [w454 w460] -> w452
              tunnel: w451 -> [w455 w463]
              tunnel: w450 -> [w454 w462]
              frame False {
              }
              frame True {
                n47 = local read "Travel per Pulse (mm)"() -> (w457:dbl)
                n48 = local read "Move Distance (mm)"() -> (w456:dbl)
                n49 = call "Sigma_MoveAbs.vi"("Direction (+)"=FALSE, "Axis (1)"=2, "error in (no error)"=w462, "Travel (1mm)"=w456, "Travel per Pulse (0.004mm)"=w457, "VISA resource name"=w463) -> ("error out"=w460:errorcluster, "VISA resource name out"=w461:refnum<visa-resource-name>)  [unwired: 4 in]
              }
            }
          }
          event "Back": Value Change {
            n50 = event-data() -> ()  [unwired: 1 in, 1 out]
            n51 = case shown="True" "Back" {
              tunnel: [w470 w476] -> w468
              tunnel: [w469 w475] -> w467
              tunnel: w466 -> [w470 w478]
              tunnel: w465 -> [w469 w477]
              frame False {
              }
              frame True {
                n52 = local read "Travel per Pulse (mm)"() -> (w472:dbl)
                n53 = local read "Move Distance (mm)"() -> (w471:dbl)
                n54 = call "Sigma_MoveAbs.vi"("Direction (+)"=TRUE, "Axis (1)"=2, "error in (no error)"=w477, "Travel (1mm)"=w471, "Travel per Pulse (0.004mm)"=w472, "VISA resource name"=w478) -> ("error out"=w475:errorcluster, "VISA resource name out"=w476:refnum<visa-resource-name>)  [unwired: 4 in]
              }
            }
          }
          event "Home X": Value Change {
            n55 = event-data() -> ()  [unwired: 1 in, 1 out]
            n56 = case shown="True" "Home X" {
              tunnel: [w485 w488] -> w480
              tunnel: [w484 w487] -> w479
              tunnel: w483 -> [w485 w490]
              tunnel: w482 -> [w484 w489]
              frame False {
              }
              frame True {
                n57 = call "Sigma_Home.vi"("Axis (1)"="1", "error in (no error)"=w489, "VISA resource name"=w490) -> ("error out"=w487:errorcluster, "VISA resource name out"=w488:refnum<visa-resource-name>)  [unwired: 7 in]
              }
            }
          }
          event "Home Y": Value Change {
            n58 = event-data() -> ()  [unwired: 1 in, 1 out]
            n59 = case shown="True" "Home Y" {
              tunnel: [w497 w500] -> w493
              tunnel: [w496 w499] -> w492
              tunnel: w495 -> [w497 w502]
              tunnel: w494 -> [w496 w501]
              frame False {
              }
              frame True {
                n60 = call "Sigma_Home.vi"("Axis (1)"="2", "error in (no error)"=w501, "VISA resource name"=w502) -> ("error out"=w499:errorcluster, "VISA resource name out"=w500:refnum<visa-resource-name>)  [unwired: 7 in]
              }
            }
          }
          event "Stop 3": Value Change {
            n61 = event-data() -> ()  [unwired: 1 in, 1 out]
            n62 = case shown="True" "Stop 3" {
              tunnel: [w509 w510] -> w507
              tunnel: [w508 w511] -> w506
              tunnel: w505 -> [w509 w513]
              tunnel: w504 -> [w508 w512]
              frame False {
              }
              frame True {
                n63 = call "Sigma_Stop.vi"("Axis (1)"="W", "error in (no error)"=w512, "VISA resource name"=w513) -> ("error out"=w511:errorcluster, "VISA resource name out"=w510:refnum<visa-resource-name>)  [unwired: 7 in]
              }
            }
          }
          event "Emergency Stop": Value Change {
            n64 = event-data() -> ()  [unwired: 1 in, 1 out]
            n65 = case shown="True" "Emergency Stop" {
              tunnel: [w521 w524] -> w519
              tunnel: [w520 w523] -> w518
              tunnel: w517 -> [w521 w526]
              tunnel: w516 -> [w520 w525]
              frame False {
              }
              frame True {
                n66 = call "Sigma_Stop.vi"("Axis (1)"="E", "error in (no error)"=w525, "VISA resource name"=w526) -> ("error out"=w523:errorcluster, "VISA resource name out"=w524:refnum<visa-resource-name>)  [unwired: 7 in]
              }
            }
          }
        }
        n67 = Unbundle By Name(w400) -> ("status"=w401:bool)
        n68 = Compound Arithmetic op=OR(w401, w397) -> (w399:bool)
      }
      n69 = call <vilib>:"Simple Error Handler.vi"("error in (no error)"=w141) -> ()  [unwired: 4 in, 5 out]
      n70 = while {
        tunnel: w121 -> [w147]
        tunnel: [w145] -> _
        tunnel: w120 -> [w146]
        tunnel: [w144] -> _
        stop <- w143 stop-if-true
        n71 = local read "Scan"() -> (w142:bool)
        n72 = case shown="True" w142 {
          selector: w142 -> [_ w186]
          tunnel: [w149 w191] -> w145
          tunnel: w147 -> [w151 w188]
          tunnel: w146 -> [w150 w187]
          tunnel: [w148 w190] -> w144
          tunnel: [FALSE w193] -> w143
          frame False {
            n73 = while {
              tunnel: w150 -> [w160]
              tunnel: [w155] -> w149
              tunnel: [w154] -> w148
              tunnel: w151 -> [w153]
              stop <- w167 stop-if-true
              # "Stop at LS"
              # "Send command and get position"
              n74 = local read "Travel per Pulse (mm)"() -> (w163:dbl)
              n75 = local read "Cur. Pos X"() -> (w157:dbl)
              n76 = local read "Cur. Pos Y"() -> (w156:dbl)
              n77 = call "Sigma_GetPos.vi"("VISA resource name"=w153, "Travel per Pulse (mm)"=w163, "Init Pos X (mm)"=w157, "Init  Pos Y (mm)"=w156, "error in (no error)"=w160) -> ("Pos X (mm)"=w159:dbl, "Pos Y (mm)"=w158:dbl, "VISA resource name out"=w162:refnum<visa-resource-name>, "State String"=w164:string, "error out"=w161:errorcluster)  [unwired: 6 in]
              n78 = local write "Cur. Pos X"(w159) -> ()
              n79 = local write "Cur. Pos Y"(w158) -> ()
              n80 = Wait Until Next ms Multiple(millisecond multiple=u32 250) -> ()  [unwired: 1 out]
              n81 = case shown="\"K\", Default" w164 {
                tunnel: [w170 w175 w180 w185] -> w155
                tunnel: [w169 w174 w179 w184] -> w154
                tunnel: w162 -> [w170 w172 w177 w182]
                tunnel: w161 -> [w169 w171 w176 w181]
                frame "K", Default {
                }
                frame "L" {
                  n82 = call "Sigma_Stop.vi"("Axis (1)"="1", "error in (no error)"=w171, "VISA resource name"=w172) -> ("error out"=w174:errorcluster, "VISA resource name out"=w175:refnum<visa-resource-name>)  [unwired: 7 in]
                }
                frame "M" {
                  n83 = call "Sigma_Stop.vi"("Axis (1)"="2", "error in (no error)"=w176, "VISA resource name"=w177) -> ("error out"=w179:errorcluster, "VISA resource name out"=w180:refnum<visa-resource-name>)  [unwired: 7 in]
                }
                frame "W" {
                  n84 = call "Sigma_Stop.vi"("Axis (1)"="W", "error in (no error)"=w181, "VISA resource name"=w182) -> ("error out"=w184:errorcluster, "VISA resource name out"=w185:refnum<visa-resource-name>)  [unwired: 7 in]
                }
              }
              n85 = Unbundle By Name(w154) -> ("status"=w168:bool)
              n86 = local read "Scan"() -> (w166:bool)
              n87 = Compound Arithmetic op=OR(w168, w166) -> (w167:bool)
            }
          }
          frame True {
            n88 = local read "Travel per Pulse (mm)"() -> (w189:dbl)
            n89 = local write "Move X"(w186) -> ()
            n90 = local read "Cur. Pos Y"() -> (w194:dbl)
            n91 = while {
              shift-right: [w214] -> _
              shift-left: TRUE ("Direction (+)") -> [w227]
              tunnel: w194 -> [w226]
              tunnel: [w222] -> w193
              tunnel: w188 -> [w229]
              tunnel: w187 -> [w228]
              tunnel: [w215] -> w191
              tunnel: [w212] -> w190
              tunnel: w189 -> [w203]
              stop <- w222 stop-if-true
              # "5. Stop scan condition"
              # "3. Run Step Y"
              # "2. wait until run to X-length"
              # "1. Move in X axis\n    Invert direction after moved Step Y"
              # "4. Update Y Possition"
              n92 = flat-sequence {
                tunnel: w229 -> [w235]
                tunnel: w228 -> [w234]
                tunnel: w227 -> [w240]
                tunnel: w226 -> [w238]
                tunnel: [w239] -> w202
                tunnel: [w233] -> w200
                tunnel: [w232] -> w198
                tunnel: [w238] -> w196
                tunnel: w203 -> [w231]
                tunnel: w202 -> [w245]
                tunnel: [w245] -> w201
                tunnel: w200 -> [w244]
                tunnel: [w244] -> w199
                tunnel: w198 -> [w243]
                tunnel: [w243] -> w197
                tunnel: w196 -> [w242]
                tunnel: [w242] -> w195
                tunnel: w201 -> [w248]
                tunnel: w199 -> [w253]
                tunnel: w197 -> [w252]
                tunnel: w195 -> [w249]
                tunnel: [w251] -> w221
                tunnel: [w250] -> w220
                tunnel: [w249] -> w216
                tunnel: [w248] -> w214
                tunnel: [w301] -> w211
                tunnel: w221 -> [w301]
                tunnel: [w300] -> w209
                tunnel: w220 -> [w300]
                tunnel: [w299] -> w207
                tunnel: w216 -> [w299]
                tunnel: w211 -> [w309]
                tunnel: [w309] -> w210
                tunnel: w209 -> [w308]
                tunnel: [w308] -> w208
                tunnel: w207 -> [w303]
                tunnel: [w304] -> w206
                tunnel: [w319] -> w225
                tunnel: [w318] -> w224
                tunnel: w210 -> [w315]
                tunnel: w208 -> [w314]
                tunnel: w206 -> [w311]
                tunnel: w225 -> [w333]
                tunnel: w224 -> [w332]
                tunnel: [w331] -> w217
                tunnel: [w330] -> w213
                tunnel: [w382] -> w219
                tunnel: [w381] -> w218
                tunnel: w217 -> [w381]
                tunnel: w213 -> [w382]
                tunnel: [w380] -> w204
                tunnel: w219 -> [w395]
                tunnel: [w396] -> w212
                tunnel: w218 -> [w396]
                tunnel: [w395] -> w215
                tunnel: [w394] -> w205
                tunnel: w204 -> [w394]
                frame #0 {
                  n93 = local read "X-length"() -> (w237:dbl)
                  n94 = local write "Move X"(FALSE ("Move X")) -> ()
                  n95 = Not(x=w240) -> (.not. x?=w239:bool)
                  n96 = call "Sigma_MoveAbs.vi"("Direction (+)"=w239, "Axis (1)"=1, "error in (no error)"=w234, "Travel (1mm)"=w237, "Travel per Pulse (0.004mm)"=w231, "VISA resource name"=w235) -> ("error out"=w232:errorcluster, "VISA resource name out"=w233:refnum<visa-resource-name>)  [unwired: 4 in]
                }
                frame #1 {
                  n97 = Wait (ms)(milliseconds to wait=10.0 ("y")) -> ()  [unwired: 1 out]
                }
                frame #2 {
                  n98 = local read "Cur. Pos X"() -> (w246:dbl)
                  n99 = local read "Cur. Pos Y"() -> (w247:dbl)
                  n100 = while {
                    tunnel: w253 -> [w266]
                    tunnel: w252 -> [w267]
                    tunnel: [w265] -> w251
                    tunnel: [w264] -> w250
                    shift-right: [w258] -> _
                    shift-left: w247 -> [w257]
                    shift-right: [w259] -> _
                    shift-left: w246 -> [w256]
                    tunnel: w246 -> [w255]
                    stop <- w274 stop-if-true
                    # "Stop at LS"
                    # "Send command and get position"
                    n101 = local read "Travel per Pulse (mm)"() -> (w270:dbl)
                    n102 = local read "X-length"() -> (w262:dbl)
                    n103 = Wait Until Next ms Multiple(millisecond multiple=u32 100) -> ()  [unwired: 1 out]
                    n104 = call "Sigma_GetPos.vi"("VISA resource name"=w266, "Travel per Pulse (mm)"=w270, "Init Pos X (mm)"=w256, "Init  Pos Y (mm)"=w257, "error in (no error)"=w267) -> ("Pos X (mm)"=w259:dbl, "Pos Y (mm)"=w258:dbl, "VISA resource name out"=w269:refnum<visa-resource-name>, "State String"=w271:string, "error out"=w268:errorcluster)  [unwired: 6 in]
                    n105 = Subtract(x=w255, y=w259) -> (x-y=w261:dbl)
                    n106 = local write "Cur. Pos X"(w259) -> ()
                    n107 = local write "Cur. Pos Y"(w258) -> ()
                    n108 = local write "Move X"(TRUE ("Move X")) -> ()
                    n109 = Absolute Value(x=w261) -> (abs(x)=w263:dbl)
                    n110 = Greater Or Equal?(x=w263, y=w262) -> (x >= y?=w260:bool)
                    n111 = local read "Stop Scan"() -> (w273:bool)
                    n112 = case shown="\"K\", Default" w271 {
                      tunnel: [w277 w282 w287 w292] -> w265
                      tunnel: [w276 w281 w286 w291] -> w264
                      tunnel: w269 -> [w277 w279 w284 w289]
                      tunnel: w268 -> [w276 w278 w283 w288]
                      frame "K", Default {
                      }
                      frame "L" {
                        n113 = call "Sigma_Stop.vi"("Axis (1)"="1", "error in (no error)"=w278, "VISA resource name"=w279) -> ("error out"=w281:errorcluster, "VISA resource name out"=w282:refnum<visa-resource-name>)  [unwired: 7 in]
                      }
                      frame "M" {
                        n114 = call "Sigma_Stop.vi"("Axis (1)"="2", "error in (no error)"=w283, "VISA resource name"=w284) -> ("error out"=w286:errorcluster, "VISA resource name out"=w287:refnum<visa-resource-name>)  [unwired: 7 in]
                      }
                      frame "W" {
                        n115 = call "Sigma_Stop.vi"("Axis (1)"="W", "error in (no error)"=w288, "VISA resource name"=w289) -> ("error out"=w291:errorcluster, "VISA resource name out"=w292:refnum<visa-resource-name>)  [unwired: 7 in]
                      }
                    }
                    n116 = Unbundle By Name(w264) -> ("status"=w275:bool)
                    n117 = Compound Arithmetic op=OR(w275, w273, w260) -> (w274:bool)
                  }
                }
                frame #3 {
                  n118 = local read "1 Rate"() -> (w297:dbl)
                  n119 = local read "Travel per Pulse (mm)"() -> (w298:dbl)
                  n120 = local write "Move X"(FALSE ("Move X")) -> ()
                  n121 = Divide(x=w297, y=w298) -> (x/y=w294:dbl)
                  n122 = Add(x=w294, y=100.0) -> (x+y=w296:dbl)
                  n123 = Wait (ms)(milliseconds to wait=w296) -> ()  [unwired: 1 out]
                }
                frame #4 {
                  n124 = local read "Y-length"() -> (w302:dbl)
                  n125 = local read "Cur. Pos Y"() -> (w307:dbl)
                  n126 = Subtract(x=w307, y=w303) -> (x-y=w306:dbl)
                  n127 = Absolute Value(x=w306) -> (abs(x)=w305:dbl)
                  n128 = Greater Or Equal?(x=w305, y=w302) -> (x >= y?=w304:bool)
                }
                frame #5 {
                  # "Stop Y"
                  n129 = local read "Step Y"() -> (w317:dbl)
                  n130 = local read "Y-length"() -> (w316:dbl)
                  n131 = local read "Stop Scan"() -> (w313:bool)
                  n132 = Greater Or Equal?(x=w317, y=w316) -> (x >= y?=w312:bool)
                  n133 = Compound Arithmetic op=OR(w311, w312, w313) -> (w310:bool)
                  n134 = case shown="False" w310 {
                    tunnel: [w324 w329] -> w319
                    tunnel: [w323 w328] -> w318
                    tunnel: w315 -> [w321 w329]
                    tunnel: w314 -> [w320 w328]
                    frame False {
                      n135 = local read "Travel per Pulse (mm)"() -> (w322:dbl)
                      n136 = local read "Step Y"() -> (w326:dbl)
                      n137 = call "Sigma_MoveAbs.vi"("Axis (1)"=2, "error in (no error)"=w320, "Travel (1mm)"=w326, "Travel per Pulse (0.004mm)"=w322, "VISA resource name"=w321) -> ("error out"=w323:errorcluster, "VISA resource name out"=w324:refnum<visa-resource-name>)  [unwired: 5 in]
                    }
                    frame True {
                      n138 = local write "Stop Scan"(TRUE ("Stop Scan")) -> ()
                    }
                  }
                }
                frame #6 {
                  n139 = disable-structure shown="Disabled" {
                    disable-tunnel: w333 -> [w339 w379]
                    disable-tunnel: w332 -> [w338 w378]
                    disable-tunnel: [w337 w378] -> w331
                    disable-tunnel: [w336 w379] -> w330
                    frame Disabled {
                      n140 = local read item#-1() -> (w335)
                      n141 = local read item#-1() -> (w334)
                      n142 = while {
                        tunnel: w339 -> [w351]
                        tunnel: w338 -> [w352]
                        tunnel: [w350] -> w336
                        tunnel: [w349] -> w337
                        shift-right: [w344] -> _
                        shift-left: w334 -> [w341]
                        shift-right: [w343] -> _
                        shift-left: w335 -> [w342]
                        tunnel: w334 -> [w340]
                        stop <- w359 stop-if-true
                        # "Stop at LS"
                        # "Send command and get position"
                        n143 = local read item#-1() -> (w355)
                        n144 = Wait Until Next ms Multiple(millisecond multiple=u32 100) -> ()  [unwired: 1 out]
                        n145 = local read item#-1() -> (w347)
                        n146 = call "Sigma_GetPos.vi"("VISA resource name"=w351, "Travel per Pulse (mm)"=w355, "Init Pos X (mm)"=w342, "Init  Pos Y (mm)"=w341, "error in (no error)"=w352) -> ("Pos X (mm)"=w343:dbl, "Pos Y (mm)"=w344:dbl, "VISA resource name out"=w354:refnum<visa-resource-name>, "State String"=w356:string, "error out"=w353:errorcluster)  [unwired: 6 in]
                        n147 = Subtract(x=w340, y=w344) -> (x-y=w346:dbl)
                        n148 = local write item#-1(w343) -> ()
                        n149 = local write item#-1(w344) -> ()
                        n150 = Absolute Value(x=w346) -> (abs(x)=w348:dbl)
                        n151 = Greater Or Equal?(x=w348, y=w347) -> (x >= y?=w345:bool)
                        n152 = local read "Stop Scan 2"() -> (w358:bool)
                        n153 = case shown="\"K\", Default" w356 {
                          tunnel: [w362 w367 w372 w377] -> w350
                          tunnel: [w361 w366 w371 w376] -> w349
                          tunnel: w354 -> [w362 w364 w369 w374]
                          tunnel: w353 -> [w361 w363 w368 w373]
                          frame "K", Default {
                          }
                          frame "L" {
                            n154 = call "Sigma_Stop.vi"("Axis (1)"="1", "error in (no error)"=w363, "VISA resource name"=w364) -> ("error out"=w366:errorcluster, "VISA resource name out"=w367:refnum<visa-resource-name>)  [unwired: 7 in]
                          }
                          frame "M" {
                            n155 = call "Sigma_Stop.vi"("Axis (1)"="2", "error in (no error)"=w368, "VISA resource name"=w369) -> ("error out"=w371:errorcluster, "VISA resource name out"=w372:refnum<visa-resource-name>)  [unwired: 7 in]
                          }
                          frame "W" {
                            n156 = call "Sigma_Stop.vi"("Axis (1)"="W", "error in (no error)"=w373, "VISA resource name"=w374) -> ("error out"=w376:errorcluster, "VISA resource name out"=w377:refnum<visa-resource-name>)  [unwired: 7 in]
                          }
                        }
                        n157 = Unbundle By Name(w349) -> ("status"=w360:bool)
                        n158 = Compound Arithmetic op=OR(w360, w358, w345) -> (w359:bool)
                      }
                    }
                    frame Enabled {
                    }
                  }
                }
                frame #7 {
                  n159 = local read "Stop Scan"() -> (w380:bool)
                }
                frame #8 {
                  # "waiting for stop speed\naxis 2 + 100ms more"
                  n160 = local read "2 Rate"() -> (w386:dbl)
                  n161 = local read "2 Max"() -> (w392:dbl)
                  n162 = local read "Travel per Pulse (mm)"() -> (w385:dbl)
                  n163 = local read "Step Y"() -> (w393:dbl)
                  n164 = Compound Arithmetic op=MULTIPLY(w386, invert w385, 2.0 ("value")) -> (w383:dbl)
                  n165 = Compound Arithmetic op=MULTIPLY(w393, invert w392, 1000.0 ("value")) -> (w390:dbl)
                  n166 = Add(x=w383, y=w390) -> (x+y=w389:dbl)
                  n167 = Add(x=w389, y=100.0) -> (x+y=w387:dbl)
                  n168 = Wait (ms)(milliseconds to wait=w387) -> ()  [unwired: 1 out]
                }
              }
              n169 = Unbundle By Name(w212) -> ("status"=w223:bool)
              n170 = Compound Arithmetic op=OR(w223, w205) -> (w222:bool)
            }
          }
        }
      }
      n171 = call <vilib>:"Simple Error Handler.vi"() -> ()  [unwired: 5 in, 5 out]
    }
    frame Enabled {
    }
  }
  n172 = flat-sequence {
    tunnel: [w548] -> w16
    frame #0 {
      n173 = call "File Dialog"("prompt"="Choose New File For Recording\n" ("button label"), "default name"="PECT_default", "pattern (all files)"="*.tdms") -> ("selected path"=w532:path, "exists"=w527:bool, "cancelled"=w528:bool)  [unwired: 9 in, 1 out]
      n174 = case shown="False" w528 {
        tunnel: w532 -> [w533 _]
        tunnel: w527 -> [w534 _]
        frame False {
          n175 = case shown="True" w534 {
            tunnel: w533 -> [w535 w536]
            frame False {
              n176 = local write "Record path"(w535) -> ()
            }
            frame True {
              n177 = Two Button Dialog(message="Existing File\nDo you want to Replace?", 1:"No" ("F button name (\"Cancel\")"), 2:"Replace" ("T button name (\"OK\")")) -> (T button?=w537:bool)
              n178 = case shown="True" w537 {
                tunnel: w536 -> [_ w545]
                tunnel: [path "" ("deleted path") w544] -> w538
                frame False {
                  n179 = local write "Stop Scan 4"(TRUE ("Exit")) -> ()
                }
                frame True {
                  n180 = Delete(path (use dialog)=w545) -> (deleted path=w544:path)  [unwired: 4 in, 2 out]
                }
              }
              "Record path" <- w538
            }
          }
        }
        frame True {
          n181 = local write "Stop Scan 4"(TRUE ("Exit")) -> ()
        }
      }
    }
    frame #1 {
      n182 = local read "Record path"() -> (w547:path)
      n183 = TDMS Open(6:FALSE ("disable buffering (T)"), 10:T5."create or replace" ("operation"), 11:w547) -> (3:w548:refnum<k34>)  [unwired: 4 in, 1 out]
    }
  }
  n184 = while {
    shift-right: [w557] -> _
    shift-left: w25 -> [w556]
    shift-right: [w553] -> _
    shift-left: w24 -> [w555]
    stop <- w552 stop-if-true
    n185 = event shown="[4] \"Home\": Value Change" {
      selector: _ -> [_ _ _ _ _ _]
      dyn-events: _ -> [_ _ _ _ _ _]
      timeout: _ -> [_ _ _ _ _ _]
      tunnel: w556 -> [w561 w575 w578 w592 w608 w628]
      tunnel: w555 -> [w560 w574 w577 w591 w607 w627]
      tunnel: [w559 w572 w580 w594 w605 w630] -> w557
      tunnel: [w558 w573 w579 w593 w604 w629] -> w553
      tunnel: ["Stop Scan 3" _ _ _ _ _] -> w551
      event "Stop Scan 3": Value Change {
        n186 = event-data() -> ()  [unwired: 1 in, 5 out]
        n187 = case shown="True" "Stop Scan 3" {
          tunnel: [w564 w567] -> w559
          tunnel: [w563 w568] -> w558
          tunnel: w561 -> [w564 w566]
          tunnel: w560 -> [w563 w565]
          frame False {
          }
          frame True {
            n188 = call "Autonics_Stop.vi"("error in (no error)"=w565, "VISA resource name"=w566) -> ("error out"=w568:errorcluster, "VISA resource name out"=w567:refnum<visa-resource-name>)  [unwired: 8 in]
          }
        }
      }
      event "Speed": Value Change {
        n189 = event-data() -> ()  [unwired: 1 in, 1 out]
        n190 = local read "Travel per  Pulse"() -> (w570:dbl)
        n191 = local read "Speed"() -> (w569:dbl)
        n192 = local read "Multiplier"() -> (w571:dbl)
        n193 = call "Autonics_Speed.vi"("Multiplier"=w571, "Speed (mm/s)"=w569, "error in (no error)"=w574, "Travel per  Pulse"=w570, "VISA resource name"=w575) -> ("error out"=w573:errorcluster, "VISA resource name out"=w572:refnum<visa-resource-name>)  [unwired: 5 in]
      }
      event "Left_": Value Change {
        n194 = event-data() -> ()  [unwired: 1 in, 1 out]
        n195 = case shown="True" "Left_" {
          tunnel: [w581 w587] -> w580
          tunnel: [w582 w586] -> w579
          tunnel: w578 -> [w581 w589]
          tunnel: w577 -> [w582 w588]
          frame False {
          }
          frame True {
            n196 = local read "Move Distance (mm) 2"() -> (w585:dbl)
            n197 = local read "Travel per  Pulse"() -> (w583:dbl)
            n198 = call "Autonics_Move.vi"("Direction (+)"="+", "error in (no error)"=w588, "Travel per Pulse (mm)"=w583, "Move Distance (mm)"=w585, "VISA resource name"=w589) -> ("error out"=w586:errorcluster, "VISA resource name out"=w587:refnum<visa-resource-name>)  [unwired: 5 in]
          }
        }
      }
      event "Right_": Value Change {
        n199 = event-data() -> ()  [unwired: 1 in, 1 out]
        n200 = case shown="True" "Right_" {
          tunnel: [w596 w601] -> w594
          tunnel: [w595 w600] -> w593
          tunnel: w592 -> [w596 w603]
          tunnel: w591 -> [w595 w602]
          frame False {
          }
          frame True {
            # "Moving distance"
            n201 = local read "Move Distance (mm) 2"() -> (w598:dbl)
            n202 = local read "Travel per  Pulse"() -> (w597:dbl)
            n203 = call "Autonics_Move.vi"("Direction (+)"="-", "error in (no error)"=w602, "Travel per Pulse (mm)"=w597, "Move Distance (mm)"=w598, "VISA resource name"=w603) -> ("error out"=w600:errorcluster, "VISA resource name out"=w601:refnum<visa-resource-name>)  [unwired: 5 in]
          }
        }
      }
      event "Home": Value Change {
        n204 = event-data() -> ()  [unwired: 1 in, 1 out]
        n205 = case shown="True" "Home" {
          tunnel: [w610 w612] -> w605
          tunnel: [w609 w611] -> w604
          tunnel: w608 -> [w610 w616]
          tunnel: w607 -> [w609 w615]
          frame False {
          }
          frame True {
            n206 = call "Autonics_Home.vi"("error in (no error)"=w615, "VISA resource name"=w616) -> ("error out"=w613:errorcluster, "VISA resource name out"=w614:refnum<visa-resource-name>)  [unwired: 8 in]
            n207 = disable-structure shown="Enabled" {
              disable-tunnel: w614 -> [w622 w625]
              disable-tunnel: w613 -> [w621 w624]
              disable-tunnel: [w620 w625] -> w612
              disable-tunnel: [w619 w624] -> w611
              frame Disabled {
                n208 = local read "Travel per  Pulse"() -> (w618:dbl)
                n209 = local read "Multiplier"() -> (w617:dbl)
                n210 = local read "Speed"() -> (w623:dbl)
                n211 = call "Autonics_Speed.vi"("Multiplier"=w617, "Speed (mm/s)"=w623, "error in (no error)"=w621, "Travel per  Pulse"=w618, "VISA resource name"=w622) -> ("error out"=w619:errorcluster, "VISA resource name out"=w620:refnum<visa-resource-name>)  [unwired: 5 in]
              }
              frame Enabled {
              }
            }
          }
        }
      }
      event "Stop motor": Value Change {
        n212 = event-data() -> ()  [unwired: 1 in, 1 out]
        n213 = case shown="True" "Stop motor" {
          tunnel: [w632 w633] -> w630
          tunnel: [w631 w636] -> w629
          tunnel: w628 -> [w632 w635]
          tunnel: w627 -> [w631 w634]
          frame False {
          }
          frame True {
            n214 = call "Autonics_Stop.vi"("error in (no error)"=w634, "VISA resource name"=w635) -> ("error out"=w636:errorcluster, "VISA resource name out"=w633:refnum<visa-resource-name>)  [unwired: 8 in]
          }
        }
      }
    }
    n215 = Unbundle By Name(w553) -> ("status"=w554:bool)
    n216 = Compound Arithmetic op=OR(w554, w551) -> (w552:bool)
  }
  n217 = while {
    shift-right: [w641] -> w31
    shift-left: w25 -> [w643]
    shift-right: [w640] -> w30
    shift-left: w24 -> [w642]
    stop <- w644 stop-if-true
    n218 = local read "Travel per  Pulse"() -> (w637:dbl)
    n219 = call "Autonics_GetPos.vi"("error in (no error)"=w642, "Travel per Pulse (mm)"=w637, "VISA resource name"=w643) -> ("error out"=w640:errorcluster, "Current  Position (mm)"=w639:dbl, "VISA resource name out"=w641:refnum<visa-resource-name>)  [unwired: 6 in]
    n220 = Wait Until Next ms Multiple(millisecond multiple=u32 100) -> ()  [unwired: 1 out]
    n221 = local write "Current  Position (mm)"(w639) -> ()
    n222 = local read "Stop Scan 3"() -> (w645:bool)
    n223 = Unbundle By Name(w640) -> ("status"=w638:bool)
    n224 = Compound Arithmetic op=OR(w638, w645) -> (w644:bool)
  }
  n225 = Unbundle By Name(w5) -> ("Frequency"=w2:dbl)
  n226 = Quotient & Remainder(x="Sample Rate", y=w2) -> (floor(x/y)=w1:dbl)  [unwired: 1 out]
  "Number of Samples 2" <- w1
  n227 = call-poly <vilib>:"DAQmx Timing.vi"("task/channels in"=w93, "sample mode"=w58, "samples per channel"=w1, "rate"="Sample Rate", "source"="Sample Clock Source 2", "error in"=w94) -> ("task out"=w96:refnum<k21>, "error out"=w95:errorcluster)  [unwired: 8 in]
  n228 = property class="DAQmx Timing"(reference=w96, error in=w95) -> (reference out=w11:refnum<k21>, error out=w10:errorcluster, "SampClk.Rate"=→"Actual Sample Rate":dbl)
  n229 = local read "Output 2D"() -> (w6:dbl[][])
  n230 = local read "Simulation"() -> (w7:bool)
  n231 = local read "Output Array"() -> (w54:T2)
  n232 = call "TDMS_Open.vi"("Gate 1"=w6, "Open"="Open 2") -> ("Output 2D"=→"Output 2D":dbl[][])  [unwired: 8 in, 1 out]
  n233 = local write "Move X"(w34) -> ()
  n234 = local write "Scan"(w34) -> ()
  n235 = case shown="True" w7 {
    tunnel: [w650 w657] -> w36
    tunnel: [w649 w656] -> w35
    tunnel: w11 -> [w648 w657]
    tunnel: w10 -> [w647 w656]
    frame False {
      n236 = call-poly <vilib>:"DAQmx Trigger.vi"("task/channels in"=w648, "source"="Digital Trigger Source", "edge"="Edge", "error in"=w647) -> ("task out"=w653:refnum<k21>, "error out"=w652:errorcluster)  [unwired: 10 in]
      n237 = property class="DAQmx Trigger"(reference=w653, error in=w652, "Start.Retriggerable"=TRUE) -> (reference out=w650:refnum<k21>, error out=w649:errorcluster)
    }
    frame True {
    }
  }
  n238 = Index Array(array=w54) -> (element=w53:T4)  [unwired: 1 in]
  n239 = VISA Close(VISA resource name=w31, error in (no error)=w30) -> ()  [unwired: 1 out]
  n240 = Unbundle By Name(w53) -> ("Frequency"=w15:dbl)
  n241 = local read "Distance_"() -> (w14:dbl)
  n242 = Divide(x="Sample Rate", y=w15) -> (x/y=w52:dbl)
  n243 = Divide(x=w52, y=2.0) -> (x/y=w50:dbl)
  n244 = call-poly <vilib>:"DAQmx Create Virtual Channel.vi"("maximum value"="Max Voltage 2", "minimum value"="Min Voltage 2", "physical channels"="Physical Channel(s)", "error in"=w35) -> ("task out"=w79:refnum<k21>, "error out"=w80:errorcluster)  [unwired: 10 in]
  n245 = Build Array(w15, "Sample Rate", w14, 1.0 ("element")) -> (w18:dbl[])
  n246 = local read "Y-length"() -> (w40:dbl)
  n247 = local read "Step Y"() -> (w41:dbl)
  n248 = TDMS Write(0:w16, 5:"Freq_Sampling_SizeX_SizeY" ("group name in (Untitled)"), 9:w18) -> (4:w12:refnum<k34>)  [unwired: 3 in, 3 out]
  n249 = Obtain Queue(max queue size (-1, unlimited)=10000, name (unnamed)="data DAQ", element data type=dbl[] [] ("data")) -> (queue out=w46:refnum<queue>)  [unwired: 2 in, 2 out]
  n250 = Quotient & Remainder(x=w40, y=w41) -> (floor(x/y)=w39:dbl)  [unwired: 1 out]
  n251 = Initialize Array(0.0 ("element"), w1) -> (w47:dbl[])
  n252 = Obtain Queue(max queue size (-1, unlimited)=10000, name (unnamed)="data Extraction", element data type=0.0) -> (queue out=w44:refnum<queue>)  [unwired: 2 in, 2 out]
  n253 = while {
    shift-right: [w658] -> _
    shift-left: T3."No Scan" -> [w672]
    shift-right: [w671] -> _
    shift-left: w25 -> [w670]
    shift-right: [w668] -> _
    shift-left: w24 -> [w669]
    shift-right: [w664] -> _
    shift-left: "+" ("Direction (+)") -> [w661]
    shift-right: [w663] -> _
    shift-left: 0.0 ("Current  Position (mm)") -> [w659]
    shift-right: [w662] -> _
    shift-left: 0.0 ("Move Distance (mm) 2") -> [w660]
    stop <- w665 stop-if-true
    n254 = case shown="\"No Scan\", Default" w672 {
      selector: w672 -> [w674 _ _]
      tunnel: [w684 w703 w710] -> w671
      tunnel: w670 -> [w684 w700 w709]
      tunnel: [w683 w702 w708] -> w668
      tunnel: w669 -> [w683 w701 w707]
      tunnel: [w682 w697 w704] -> w664
      tunnel: [w681 w698 w705] -> w663
      tunnel: [w680 w699 w706] -> w662
      tunnel: w661 -> [w675 w697 w704]
      tunnel: w660 -> [_ w699 w706]
      tunnel: w659 -> [_ w698 w705]
      tunnel: [w673 T3."Wait to destination X" w711] -> w658
      frame "No Scan", Default {
        n255 = local read "Current  Position (mm)"() -> (w681:dbl)
        n256 = local read "Distance_"() -> (w680:dbl)
        n257 = Build Array("Left 3", "Right 3") -> (w677:bool[])
        n258 = Boolean Array To Number(Boolean array=w677) -> (number=w676:u32)
        n259 = case shown="0, Default" w676 {
          tunnel: [w688 "-" ("Direction (+)") "+" ("Direction (+)")] -> w682
          tunnel: w675 -> [w688 _ _]
          tunnel: w674 -> [w686 _ _]
          tunnel: [w686 T3."Scan X" T3."Scan X"] -> w673
          frame 0, Default {
            w687 = FALSE ("Scan")
            n260 = Wait (ms)(milliseconds to wait=u32 100) -> ()  [unwired: 1 out]
            n261 = local write "Scan"(w687) -> ()
            n262 = local write "Move X"(w687) -> ()
          }
          frame 1 {
            w690 = TRUE ("Scan")
            n263 = local write "Scan"(w690) -> ()
            n264 = local write "Move X"(w690) -> ()
          }
          frame 2 {
            w693 = TRUE ("Scan")
            n265 = local write "Scan"(w693) -> ()
            n266 = local write "Move X"(w693) -> ()
          }
        }
      }
      frame "Scan X" {
        n267 = local read "Travel per  Pulse"() -> (w695:dbl)
        n268 = call "Autonics_Move.vi"("Direction (+)"=w697, "error in (no error)"=w701, "Travel per Pulse (mm)"=w695, "Move Distance (mm)"=w699, "VISA resource name"=w700) -> ("error out"=w702:errorcluster, "VISA resource name out"=w703:refnum<visa-resource-name>)  [unwired: 5 in]
      }
      frame "Wait to destination X" {
        n269 = local read "Current  Position (mm)"() -> (w713:dbl)
        n270 = Absolute Value(x=w706) -> (abs(x)=w718:dbl)
        n271 = Subtract(x=w713, y=w705) -> (x-y=w714:dbl)
        n272 = Absolute Value(x=w714) -> (abs(x)=w717:dbl)
        n273 = Subtract(x=w717, y=w718) -> (x-y=w720:dbl)
        n274 = Number To Fractional String(number=w720, precision (6)=i16 1 ("정밀도(6)")) -> (F-format string=w715:string)  [unwired: 2 in]
        n275 = Fract/Exp String To Number(string=w715) -> (number=w719:dbl)  [unwired: 3 in, 1 out]
        n276 = Less Than 0?(x=w719) -> (x < 0?=w712:bool)
        n277 = case shown="False" w712 {
          tunnel: [T3."No Scan" T3."Wait to destination X"] -> w711
          tunnel: [w723 w726] -> w710
          tunnel: w709 -> [w723 w726]
          tunnel: [w722 w725] -> w708
          tunnel: w707 -> [w722 w725]
          frame False {
            w721 = FALSE ("Left 3")
            n278 = local write "Left 3"(w721) -> ()
            n279 = local write "Right 3"(w721) -> ()
          }
          frame True {
            n280 = Wait Until Next ms Multiple(millisecond multiple=u32 100) -> ()  [unwired: 1 out]
          }
        }
      }
    }
    n281 = local read "Stop Scan 3"() -> (w667:bool)
    n282 = Unbundle By Name(w668) -> ("status"=w666:bool)
    n283 = Compound Arithmetic op=OR(w666, w667) -> (w665:bool)
  }
  n284 = case shown="\"                    Test mode                   \"" "Tab Control 2" {
    tunnel: w36 -> [w733 w946]
    tunnel: [w746 w940] -> w85
    tunnel: [w745 w939] -> w84
    tunnel: w47 -> [w743 w948]
    tunnel: w35 -> [w732 w945]
    tunnel: w50 -> [w744 w947]
    tunnel: w46 -> [w742 _]
    tunnel: w44 -> [w741 _]
    tunnel: w39 -> [w736 _]
    tunnel: w12 -> [w729 _]
    frame "                          Scan mode                      ", Default {
      # "Column"
      # "Row"
      n285 = To Long Integer(number=w736) -> (32bit integer=w731:i32)
      n286 = disable-structure shown="Disabled" {
        frame Disabled {
          n287 = Decrement() -> (x-1=w749:dbl)  [unwired: 1 in]
          n288 = Decrement() -> (x-1=w748:dbl)  [unwired: 1 in]
          n289 = call "Surface_AxesScale.vi"("Y-axis Max"=w748, "X-axis max"=w749, "Auto Scale"=FALSE) -> ()  [unwired: 9 in]
        }
        frame Enabled {
        }
      }
      n290 = Increment(x=w731) -> (x+1=w730:i32)
      n291 = while {
        stop <- w766 stop-if-true
        n292 = local read "Out Array"() -> (w750:dbl[][])
        n293 = call "CSV Save.vi"("Array"=w750, "Save Button"="Save Scan mode") -> ()  [unwired: 9 in, 1 out]
        n294 = Delete From Array(array=w750, length=1 ("길이"), index (row)=0 ("인덱스 (행)")) -> (array with subset deleted=w759:dbl[][])  [unwired: 1 in, 1 out]
        n295 = disable-structure shown="비활성화" {
          disable-tunnel: w750 -> [w768 _]
          frame Disabled {
            n296 = call <vilib>:"3D Surface.vi"("z matrix"=w768, "3D graph"="3D Surface") -> ()  [unwired: 8 in, 2 out]
            n297 = local read "3D Surface"() -> (w772:refnum<k7>)
            n298 = property class="CWGraph3D"(reference=w772, "ViewMode"="ViewMode Analysis") -> ()  [unwired: 1 in, 2 out]
            n299 = call <vilib>:"Basic Properties.vi"("3D graph"=w772, "plot style"="Plot style Analysis") -> ()  [unwired: 12 in, 2 out]
          }
          frame Enabled {
          }
        }
        n300 = Delete From Array(array=w759, length=1 ("길이"), index (row)=0 ("인덱스 (행)")) -> (array with subset deleted=w761:dbl[][])  [unwired: 1 in, 1 out]
        n301 = Subtract ("Subtract.vi")(x=w761, y=w759) -> (x-y=w754:dbl[][])
        n302 = Wait (ms)(milliseconds to wait=u32 100) -> ()  [unwired: 1 out]
        n303 = call "Filters.vi"("filter type"=Filter_Passband_Type."Lowpass", "Order"=2.0, "Input data"=w754, "Sampling Freq"=1000.0, "Low Cutoff Freq"="Low Cutoff Freq") -> ("Filterd Data Matrix"=w753:T9)  [unwired: 10 in]
        n304 = Transpose 2D Array(2D array=w753) -> (transposed array=→"Differential data":T9)
        n305 = Transpose 2D Array(2D array=w759) -> (transposed array=→"Normal data":dbl[][])
        n306 = local read "Stop Scan"() -> (w766:bool)
      }
      n307 = while {
        shift-right: [w843] -> _
        shift-left: w743 -> [w847]
        tunnel: w743 -> [w846]
        tunnel: w744 -> [w845]
        tunnel: w742 -> [w844]
        tunnel: w741 -> [w842]
        shift-right: [w824] -> _
        shift-left: dbl[][] [] ("Out Array") -> [w841]
        shift-right: [w832] -> _
        shift-left: 0 -> [w840]
        shift-right: [w831] -> _
        shift-left: 0 -> [w836]
        shift-right: [w830] -> _
        shift-left: FALSE ("Output Direction") -> [w839]
        tunnel: w730 -> [w835]
        shift-right: [w828] -> _
        shift-left: FALSE -> [w829]
        shift-right: [w827] -> _
        shift-left: 0 -> [w826]
        tunnel: w729 -> [w823]
        stop <- w837 stop-if-true
        n308 = local read "Move X"() -> (w833:bool)
        n309 = local read "Scan"() -> (w834:bool)
        n310 = Equal?(x=w836, y=w835) -> ()  [unwired: 1 out]
        n311 = And(x=w834, y=w833) -> (x .and. y?=w828:bool)
        n312 = case shown="True" w828 {
          selector: w828 -> [w852 w881]
          tunnel: w847 -> [w859 w884]
          tunnel: w846 -> [_ w895]
          tunnel: w845 -> [_ w894]
          tunnel: w844 -> [_ w893]
          tunnel: [w859 w892] -> w843
          tunnel: w842 -> [_ w891]
          tunnel: w841 -> [w856 w890]
          tunnel: [w854 w882] -> w824
          tunnel: w840 -> [w858 w889]
          tunnel: w836 -> [w850 w888]
          tunnel: w839 -> [w857 w878]
          tunnel: [w857 w887] -> w830
          tunnel: [w858 w886] -> w832
          tunnel: [w849 w885] -> w831
          tunnel: w826 -> [w848 w876]
          tunnel: w829 -> [w853 w880]
          tunnel: [w848 w872] -> w827
          tunnel: w823 -> [_ w870]
          frame False {
            n313 = Not Equal?(x=w853, y=w852) -> (x != y?=w851:bool)
            n314 = case shown="True" w851 {
              tunnel: w850 -> [w861 w863]
              tunnel: [w861 w862] -> w849
              frame False {
              }
              frame True {
                n315 = Increment(x=w863) -> (x+1=w862:i32)
              }
            }
            n316 = disable-structure shown="비활성화" {
              frame Disabled {
                n317 = Wait (ms)(milliseconds to wait=u32 100 ("대기 시간(ms)")) -> ()  [unwired: 1 out]
              }
              frame Enabled {
              }
            }
            n318 = call "CSV Open.vi"("2D Array In"=w856, "Open"="Open") -> ("2D Array Out"=w854:dbl[][])  [unwired: 9 in]
            n319 = case shown="True" "Open" {
              tunnel: w854 -> [_ w864]
              frame False {
              }
              frame True {
                n320 = Matrix Size(0:w864) -> (1:w865:i32, 2:w866:i32)
                n321 = Decrement(x=w865) -> (x-1=w869:i32)
                n322 = Decrement(x=w866) -> (x-1=w868:i32)
                n323 = call "Surface_AxesScale.vi"("Y-axis Max"=w868, "X-axis max"=w869, "Auto Scale"=FALSE) -> ()  [unwired: 9 in]
              }
            }
          }
          frame True {
            n324 = Not Equal?(x=w881, y=w880) -> (x != y?=w879:bool)
            n325 = local read "Average"() -> (w883:i32)
            n326 = case shown="True" w879 {
              tunnel: w878 -> [w898 w900]
              tunnel: [w898 w899] -> w877
              frame False {
              }
              frame True {
                n327 = Not(x=w900) -> (.not. x?=w899:bool)
              }
            }
            n328 = Increment(x=w876) -> (x+1=w872:i32)
            n329 = Quotient & Remainder(x=w872, y=w883) -> (x-y*floor(x/y)=w896:i32)  [unwired: 1 out]
            n330 = Dequeue Element(queue=w893) -> (element=w875:dbl[])  [unwired: 2 in, 3 out]
            n331 = Equal To 0?(x=w896) -> (x = 0?=w874:bool)
            n332 = Empty Array?(array=w875) -> (empty?=w873:bool)
            n333 = Add(x=w875, y=w884) -> (x+y=w897:dbl[])
            n334 = Compound Arithmetic op=AND(invert w873, w874) -> (w871:bool)
            n335 = case shown="True" w871 {
              tunnel: w883 -> [_ w922]
              tunnel: w897 -> [w905 w928]
              tunnel: [w905 w927] -> w892
              tunnel: w895 -> [_ w927]
              tunnel: w894 -> [_ w921]
              tunnel: w891 -> [_ w919]
              tunnel: w890 -> [w904 w916]
              tunnel: [w904 w917] -> w882
              tunnel: w889 -> [w903 w915]
              tunnel: w888 -> [w902 w914]
              tunnel: w877 -> [w901 w910]
              tunnel: [w901 w911] -> w887
              tunnel: [w903 w912] -> w886
              tunnel: [w902 w913] -> w885
              tunnel: w870 -> [_ w908]
              frame False {
              }
              frame True {
                n336 = local read "Offset"() -> (w918:bool)
                n337 = Divide(x=w928, y=w922) -> (x/y=w907:dbl[])
                n338 = case shown="True" w918 {
                  tunnel: w921 -> [_ w937]
                  tunnel: w907 -> [w929 w931]
                  tunnel: [w929 w930] -> w920
                  frame False {
                  }
                  frame True {
                    w933 = 2.0 ("y")
                    n339 = Divide(x=w937, y=w933) -> (x/y=w938:dbl)
                    n340 = Index Array(array=w931, index #2=w938) -> (element #1=w935:dbl, element #2=w936:dbl)  [unwired: 1 in]
                    n341 = Add(x=w935, y=w936) -> (x+y=w934:dbl)
                    n342 = Divide(x=w934, y=w933) -> (x/y=w932:dbl)
                    n343 = Subtract(x=w931, y=w932) -> (x-y=w930:dbl[])
                  }
                }
                n344 = TDMS Write(0:w908, 1:enum16{"decimated", "interleaved"}."decimated" ("data layout (0:decimated)"), 9:w907) -> ()  [unwired: 3 in, 4 out]
                n345 = Array Subset(array=w920, length=w921) -> (w925:dbl[])  [unwired: 1 in]
                n346 = Array Subset(array=w920, index=w921, length=w921) -> (w924:dbl[])
                n347 = Subtract(x=w925, y=w924) -> (x-y=w923:dbl[])
                n348 = Add Array Elements(numeric array=w923) -> (sum=w926:dbl)
                n349 = Divide(x=w926, y=w921) -> (x/y=w909:dbl)
                n350 = call "EletoMatr-no trigger.vi"("Input Array"=w916, "Input"=w909, "In Row"=w915, "In Column"=w914, "Input Direction"=w910) -> ("Out Array"=w917:dbl[][], "Output Direction"=w911:bool, "Out Row"=w912:i32, "Out Column"=w913:i32)  [unwired: 7 in]
                n351 = disable-structure shown="Disabled" {
                  frame Disabled {
                  }
                  frame Enabled {
                  }
                }
                n352 = Lossy Enqueue Element(queue=w919, element=w909) -> ()  [unwired: 1 in, 4 out]
              }
            }
          }
        }
        "Out Array" <- w824
        n353 = local read "Stop Scan"() -> (w838:bool)
        n354 = Compound Arithmetic op=OR(FALSE ("값"), w838) -> (w837:bool)
        "Y line" <- w836
      }
      n355 = while {
        tunnel: w733 -> [w775]
        tunnel: [w781] -> w746
        tunnel: [w780] -> w745
        tunnel: w732 -> [w774]
        tunnel: w742 -> [w779]
        stop <- w773 stop-if-true
        n356 = And(x="Scan", y="Move X") -> (x .and. y?=w777:bool)
        n357 = case shown="True" w777 {
          tunnel: w775 -> [w783 w792]
          tunnel: [w783 w788] -> w781
          tunnel: [w782 w785] -> w780
          tunnel: w774 -> [w782 w791]
          tunnel: w779 -> [_ w793]
          frame False {
            n358 = disable-structure shown="비활성화" {
              frame Disabled {
                n359 = Wait (ms)(milliseconds to wait=u32 100 ("대기 시간(ms)")) -> ()  [unwired: 1 out]
              }
              frame Enabled {
              }
            }
          }
          frame True {
            n360 = call <vilib>:"DAQmx Start Task.vi"("task/channels in"=w792, "error in"=w791) -> ("task out"=w790:refnum<k21>, "error out"=w789:errorcluster)  [unwired: 12 in]
            n361 = while {
              tunnel: w790 -> [w808]
              tunnel: [w807] -> w787
              tunnel: [w806] -> w786
              tunnel: w789 -> [w805]
              tunnel: w793 -> [w804]
              i -> [w796]
              stop <- w798 stop-if-true
              n362 = case shown="True" "Simulation" {
                tunnel: w808 -> [w814 w822]
                tunnel: [w813 w822] -> w807
                tunnel: [w812 w821] -> w806
                tunnel: w805 -> [w811 w821]
                tunnel: [w810 w820] -> w795
                tunnel: w796 -> [_ w817]
                tunnel: [_ w815] -> w794
                frame False {
                  n363 = call-poly <vilib>:"DAQmx Read.vi"("task/channels in"=w814, "timeout"=-1.0, "error in"=w811) -> ("task out"=w813:refnum<k21>, "data"=w810:dbl[], "error out"=w812:errorcluster)  [unwired: 10 in]
                }
                frame True {
                  n364 = local read "Sample Rate"() -> (w819:dbl)
                  n365 = local read "Number of Samples 2"() -> (w818:i32)
                  n366 = local read "Output 2D"() -> (w816:dbl[][])
                  n367 = call "DAQ simulation.vi"("Sampling rate"=w819, "Samples per channel"=w818, "index (row)"=w817, "Input data"=w816) -> ("Stop"=w815:bool, "Output"=w820:dbl[])  [unwired: 6 in]
                }
              }
              n368 = local read "Move X"() -> (w801:bool)
              n369 = local read "Scan"() -> (w800:bool)
              n370 = And(x=w800, y=w801) -> (x .and. y?=w799:bool)
              n371 = Enqueue Element At Opposite End(queue=w804, element=w795) -> ()  [unwired: 2 in, 3 out]
              n372 = local read "Stop Scan"() -> (w802:bool)
              n373 = Unbundle By Name(w806) -> ("status"=w803:bool)
              n374 = Compound Arithmetic op=OR(w794, w803, w802, invert w799) -> (w798:bool)
            }
            n375 = call <vilib>:"DAQmx Stop Task.vi"("task/channels in"=w787, "error in"=w786) -> ("task out"=w788:refnum<k21>, "error out"=w785:errorcluster)  [unwired: 12 in]
          }
        }
        n376 = local read "Stop Scan"() -> (w773:bool)
      }
    }
    frame "                    Test mode                   " {
      n377 = call <vilib>:"DAQmx Start Task.vi"("task/channels in"=w946, "error in"=w945) -> ("task out"=w944:refnum<k21>, "error out"=w943:errorcluster)  [unwired: 12 in]
      n378 = while {
        tunnel: w944 -> [w971]
        tunnel: w943 -> [w970]
        tunnel: [w967] -> w941
        tunnel: [w968] -> w942
        shift-right: [w960] -> _
        shift-left: w948 -> [w962]
        tunnel: w948 -> [w958]
        shift-right: [w956] -> _
        shift-left: _ -> [w955]
        tunnel: w947 -> [w954]
        shift-right: [w953] -> _
        shift-left: _ -> [w952]
        i -> [w959]
        stop <- w969 stop-if-true
        n379 = Quotient & Remainder(x=w959, y="Average") -> (x-y*floor(x/y)=w965:i32)  [unwired: 1 out]
        n380 = call-poly <vilib>:"DAQmx Read.vi"("task/channels in"=w971, "timeout"=-1.0, "error in"=w970) -> ("task out"=w968:refnum<k21>, "data"=w961:waveform(dbl), "error out"=w967:errorcluster)  [unwired: 10 in]
        n381 = Equal To 0?(x=w965) -> (x = 0?=w964:bool)
        n382 = Unbundle By Name(w961) -> ("Y"=w951:dbl[])
        n383 = Add(x=w951, y=w962) -> (x+y=w957:dbl[])
        n384 = case shown="True" w964 {
          tunnel: "Average" -> [_ w981]
          tunnel: w961 -> [_ w996]
          tunnel: w957 -> [w974 w995]
          tunnel: [w974 w994] -> w960
          tunnel: w958 -> [_ w994]
          tunnel: [w973 w991] -> w956
          tunnel: w955 -> [w973 w975]
          tunnel: w954 -> [_ w980]
          tunnel: [w972 w986] -> w953
          tunnel: w952 -> [w972 w988]
          frame False {
          }
          frame True {
            n385 = Divide(x=w995, y=w981) -> (x/y=w979:dbl[])
            n386 = case shown="True" "Offset" {
              tunnel: w980 -> [_ w1005]
              tunnel: w979 -> [w997 w999]
              tunnel: [w997 w998] -> w977
              frame False {
              }
              frame True {
                w1001 = 2.0 ("y")
                n387 = Divide(x=w1005, y=w1001) -> (x/y=w1006:dbl)
                n388 = Index Array(array=w999, index #2=w1006) -> (element #1=w1003:dbl, element #2=w1004:dbl)  [unwired: 1 in]
                n389 = Add(x=w1003, y=w1004) -> (x+y=w1002:dbl)
                n390 = Divide(x=w1002, y=w1001) -> (x/y=w1000:dbl)
                n391 = Subtract(x=w999, y=w1000) -> (x-y=w998:dbl[])
              }
            }
            n392 = Bundle By Name(cluster=w996, "Y"=w977) -> (w976:waveform(dbl))
            n393 = Array Subset(array=w977, length=w980) -> (w985:dbl[])  [unwired: 1 in]
            n394 = Array Subset(array=w977, index=w980, length=w980) -> (w984:dbl[])
            n395 = Subtract(x=w985, y=w984) -> (x-y=w983:dbl[])
            n396 = xnode "Spectral Measurements"("신호"=w976) -> ("PSD"=w989:cluster{"f0":dbl, "df":dbl, "magnitude":dbl[]})  [unwired: 1 in, 1 out]
            n397 = Add Array Elements(numeric array=w983) -> (sum=w990:dbl)
            n398 = Divide(x=w990, y=w980) -> (x/y=→"Feature Extraction":dbl)
            n399 = case shown="True" "2 Plots" {
              tunnel: [w1010 w1016] -> w993
              tunnel: w975 -> [_ w1015]
              tunnel: [w1009 w1015] -> w991
              tunnel: w976 -> [w1009 w1011]
              tunnel: w989 -> [w1007 w1013]
              tunnel: [w1008 w1014] -> w987
              tunnel: w988 -> [_ w1012]
              tunnel: [w1007 w1012] -> w986
              frame False {
                n400 = Build Array(w1007, w1007) -> (w1008:cluster{"f0":dbl, "df":dbl, "magnitude":dbl[]}[])
                n401 = Build Array(w1009, w1009) -> (w1010:waveform(dbl)[])
              }
              frame True {
                n402 = Build Array(w1012, w1013) -> (w1014:cluster{"f0":dbl, "df":dbl, "magnitude":dbl[]}[])
                n403 = Build Array(w1015, w1011) -> (w1016:waveform(dbl)[])
              }
            }
            "Power spectral density" <- w987
            "Hall sensors signal" <- w993
          }
        }
        n404 = local read "Stop Scan"() -> (w950:bool)
        n405 = Unbundle By Name(w967) -> ("status"=w966:bool)
        n406 = Or(x=w966, y=w950) -> (x .or. y?=w969:bool)
      }
      n407 = call <vilib>:"DAQmx Stop Task.vi"("task/channels in"=w942, "error in"=w941) -> ("task out"=w940:refnum<k21>, "error out"=w939:errorcluster)  [unwired: 12 in]
    }
  }
  n408 = call-poly <vilib>:"DAQmx Timing.vi"("task/channels in"=w79, "sample mode"=w81, "rate"="Sample Rate 2", "source"="Sample Clock Source", "error in"=w80) -> ("task out"=w83:refnum<k21>, "error out"=w82:errorcluster)  [unwired: 9 in]
  n409 = property class="DAQmx Timing"(reference=w83, error in=w82) -> (reference out=w65:refnum<k21>, error out=w69:errorcluster, "SampClk.Rate"=w67:dbl)
  "Actual Sample Rate 2" <- w67
  n410 = To Double Precision Float(number="Number of Samples") -> (double precision float=w62:dbl)
  n411 = Bundle By Name(cluster=cluster{"Fs":dbl, "#s":dbl} {"Fs"=1000.0, "#s"=1000.0} ("sampling info"), "#s"=w62, "Fs"=w67) -> (w66:cluster{"Fs":dbl, "#s":dbl})
  n412 = for {
    tunnel: w69 -> [w1034]
    tunnel: w66 -> [w1033]
    tunnel: [w1032] -> w63
    tunnel: "Output Array" -> [w1031] mode=indexing
    tunnel: [w1028] -> w60 mode=indexing
    n413 = Unbundle By Name(w1031) -> ("Waveform Type"=w1030:u16, "Frequency"=w1029:dbl, "Amplitude"=w1026:dbl)
    n414 = call <vilib>:"Basic Function Generator.vi"("square wave duty cycle (%)"="Duty cycle %", "sampling info"=w1033, "signal type"=w1030, "error in (no error)"=w1034, "amplitude"=w1026, "frequency"=w1029) -> ("error out"=w1032:errorcluster, "signal out"=w1028:waveform(dbl))  [unwired: 3 in, 1 out]
  }
  "Waveform Graph 2" <- w60
  n415 = call-poly <vilib>:"DAQmx Write.vi"("task/channels in"=w65, "data"=w60, "error in"=w63) -> ("task out"=w64:refnum<k21>, "error out"=w56:errorcluster)  [unwired: 10 in, 1 out]
  n416 = call <vilib>:"DAQmx Start Task.vi"("task/channels in"=w64, "error in"=w56) -> ("task out"=w78:refnum<k21>, "error out"=w57:errorcluster)  [unwired: 12 in]
  n417 = while {
    tunnel: w78 -> [w1043]
    tunnel: w57 -> [w1042]
    tunnel: [w1040] -> w76
    tunnel: [w1041] -> w77
    stop <- w1035 stop-if-true
    n418 = call <vilib>:"DAQmx Is Task Done.vi"("task/channels in"=w1043, "error in"=w1042) -> ("task out"=w1041:refnum<k21>, "error out"=w1040:errorcluster)  [unwired: 11 in, 1 out]
    n419 = local read "Stop Scan"() -> (w1038:bool)
    n420 = Unbundle By Name(w1040) -> ("status"=w1036:bool)
    n421 = Wait Until Next ms Multiple(millisecond multiple=u32 100) -> ()  [unwired: 1 out]
    n422 = Compound Arithmetic op=OR(w1036, "Stop", w1038) -> (w1035:bool)
  }
  n423 = call <vilib>:"DAQmx Clear Task.vi"("task in"=w77, "error in"=w76) -> ("error out"=w75:errorcluster)  [unwired: 13 in]
  n424 = call <vilib>:"Simple Error Handler.vi"("error in (no error)"=w75) -> ()  [unwired: 4 in, 5 out]
  n425 = call <vilib>:"DAQmx Clear Task.vi"("task in"=w85, "error in"=w84) -> ("error out"=w92:errorcluster)  [unwired: 13 in]
  n426 = call <vilib>:"Simple Error Handler.vi"("error in (no error)"=w92) -> ()  [unwired: 4 in, 5 out]
